vi "FixJKIHelper.vi"() -> ()   [LabVIEW 2017]
uses:
  _Support/Common/Format Timestamp.vi
  _Shared/CSM Shared.lvlib
  _csmDoc/csmdoc.lvlib
  Communicable State Machine.lvlib
  user32.dll
panel:
  out "String Cache":string
  in  "Bottom Right":string
  in  "Bottom Left":string
  out "2D Picture":picture
  in  "Error in":errorcluster caption="error in (no error)"
  out "Listbox":i32(listbox)
  in  "Progress Bar":u8(slide) scale=-1.0..291.0
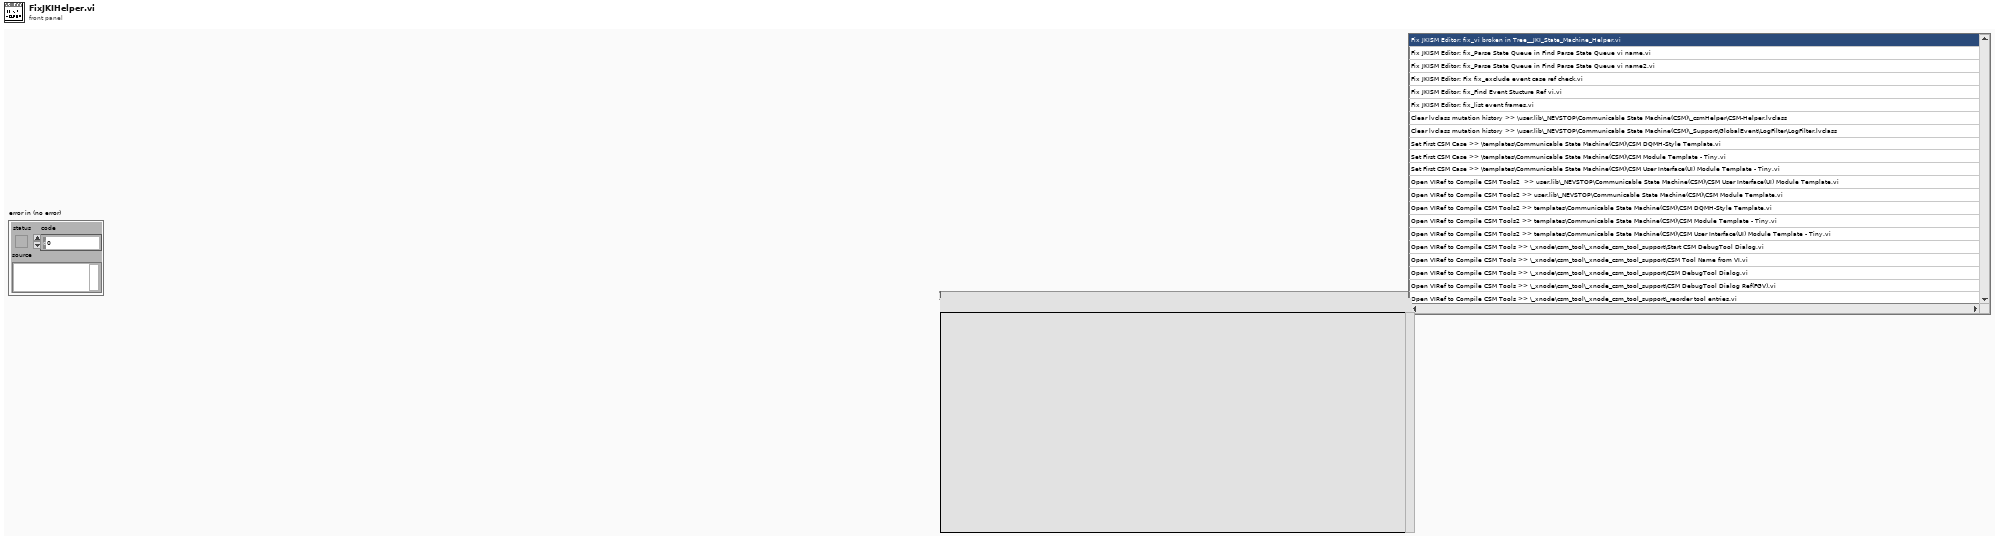
[diagram p1: front panel]
types:
  T1 = enum32{"Invalid", "Standard", "Closed", "Hidden", "Minimized", "Maximized"}
  T2 = enum32{"invalid app kind", "Development System", "Run Time System", "Student Edition", "Embedded LabVIEW", "Evaluation", "Custom"}
  T3 = cluster{"Core":cluster{"Current VI Reference":refnum<vi>, "Close Panel on Exit?":bool}, "Listbox Symbols":i32[], "Listbox Index":i32, "_JKI State Machine Helper VIs":path[], "CSM Templates":path[], "CSM lvclass":path[], "_JKI State Machine Helper Folders":path[], "Actions":string[], "LangID":string, "DescMap":variant, "NoteMap":variant, "Polish":cluster{"Version":refnum<vi>, "Action":refnum<vi>, "Progress Bar":refnum<vi>, "2D Picture":refnum<vi>, "Hold":bool, "Slides":picture[]}}
  T4 = cluster{"Version":refnum<vi>, "Action":refnum<vi>, "Progress Bar":refnum<vi>, "2D Picture":refnum<vi>, "Hold":bool, "Slides":picture[]}
  T5 = cluster{"Current VI Reference":refnum<vi>, "Close Panel on Exit?":bool}
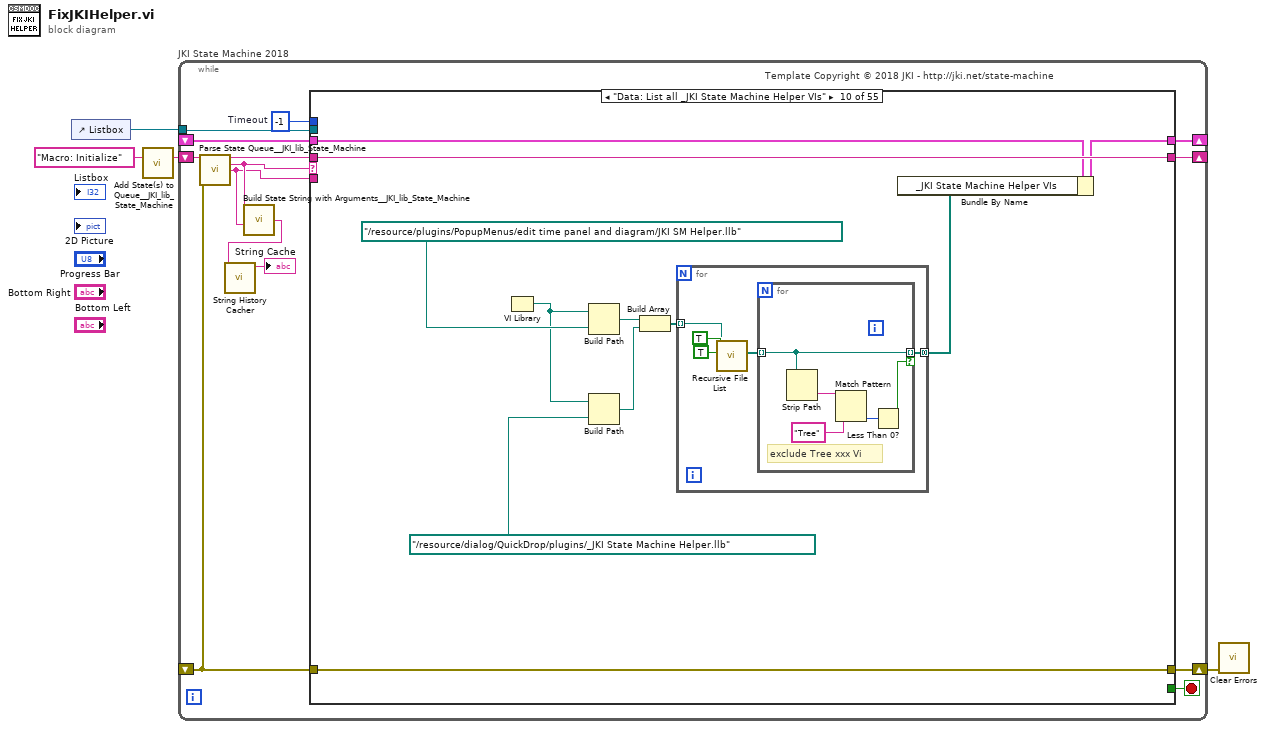
[diagram p0: block diagram]
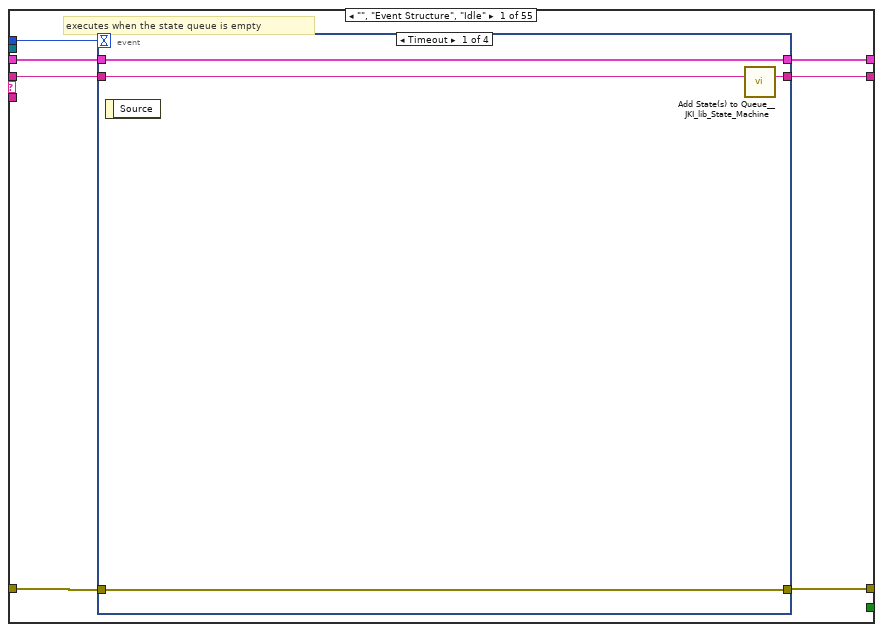
[diagram p2: hidden frame]
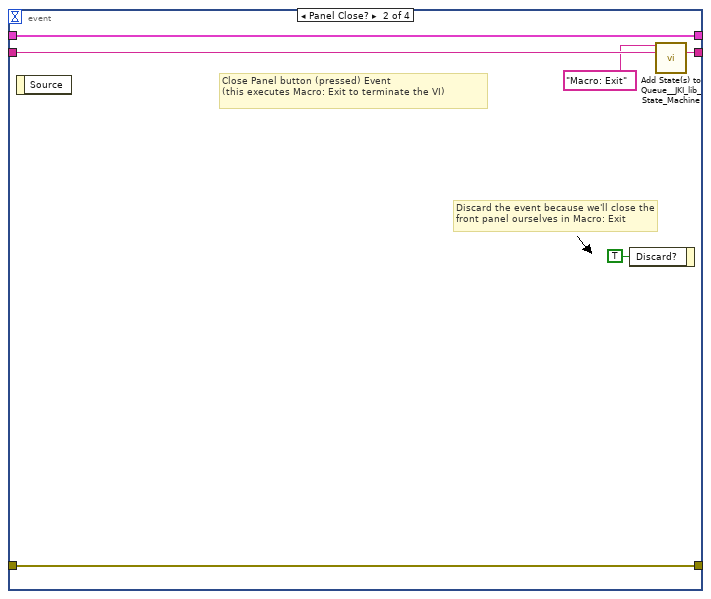
[diagram p3: hidden frame]
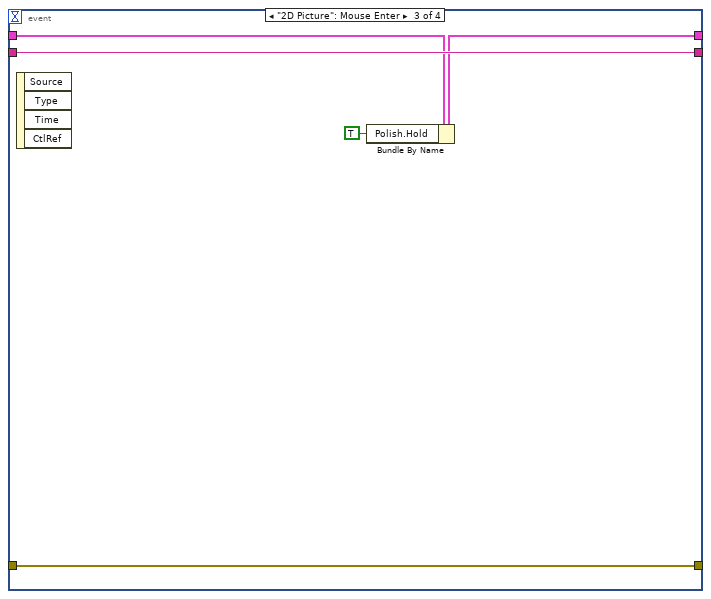
[diagram p4: hidden frame]
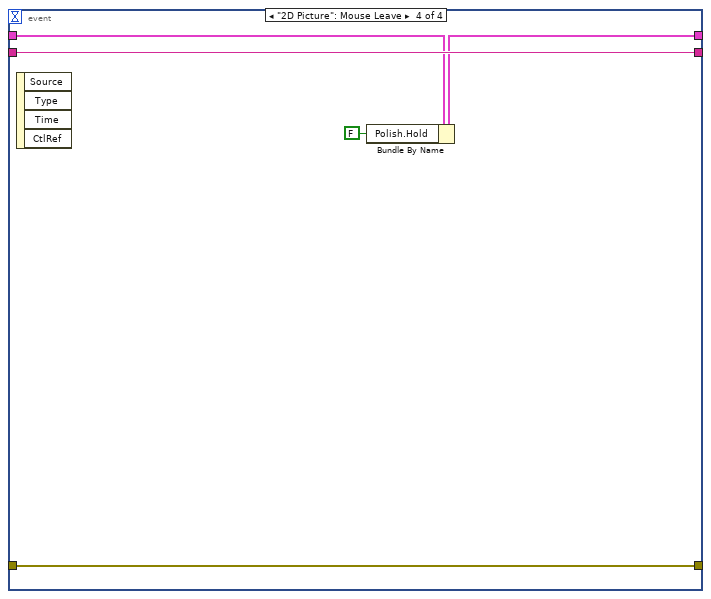
[diagram p5: hidden frame]
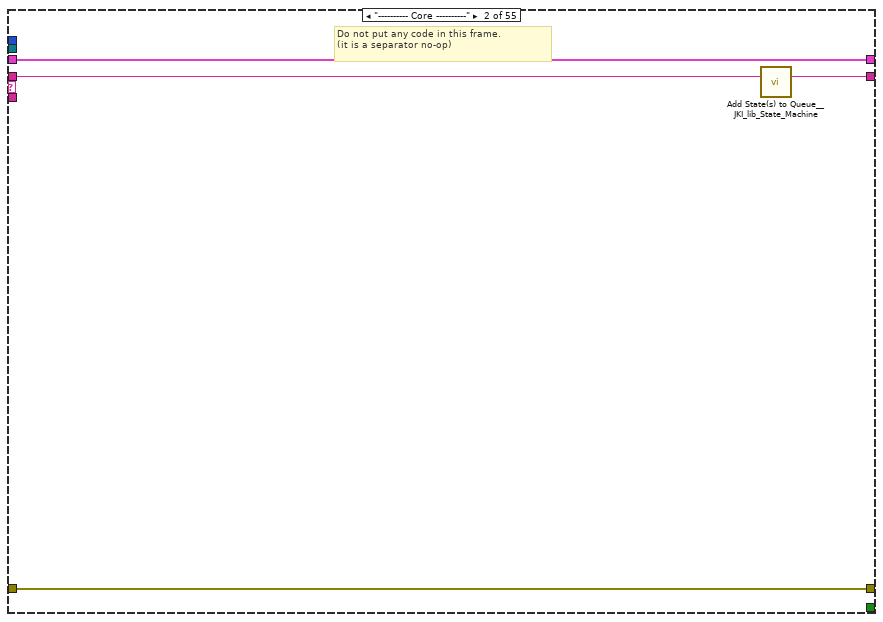
[diagram p6: hidden frame]
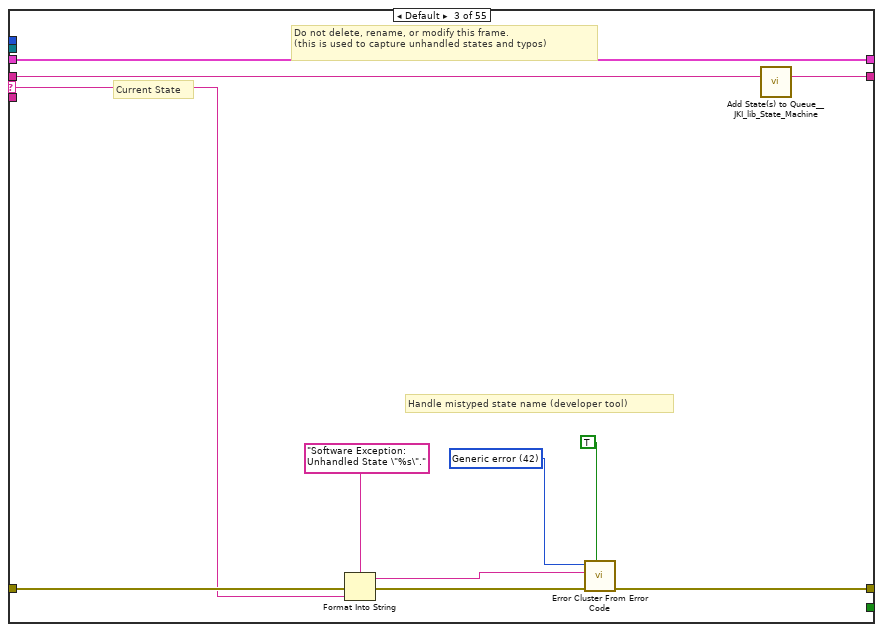
[diagram p7: hidden frame]
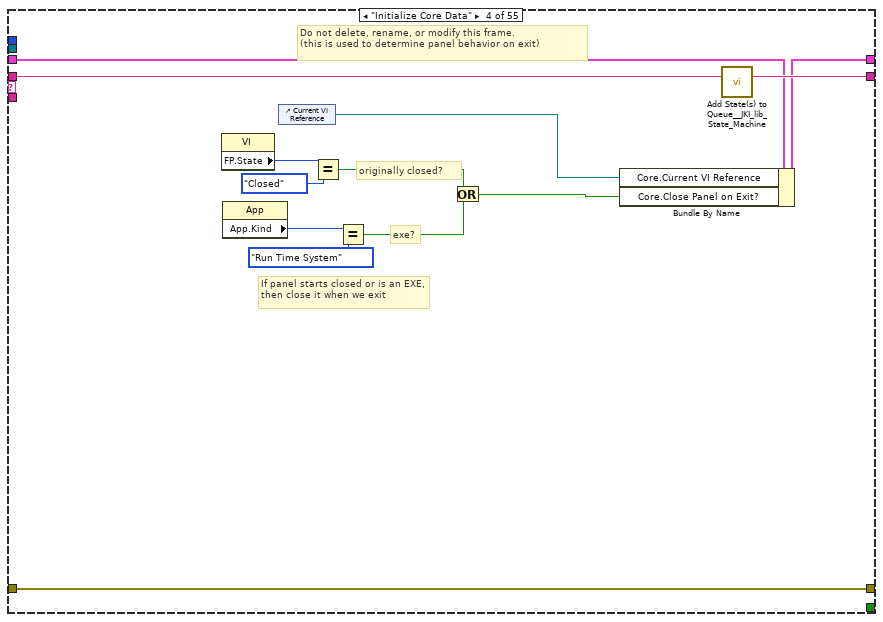
[diagram p8: hidden frame]
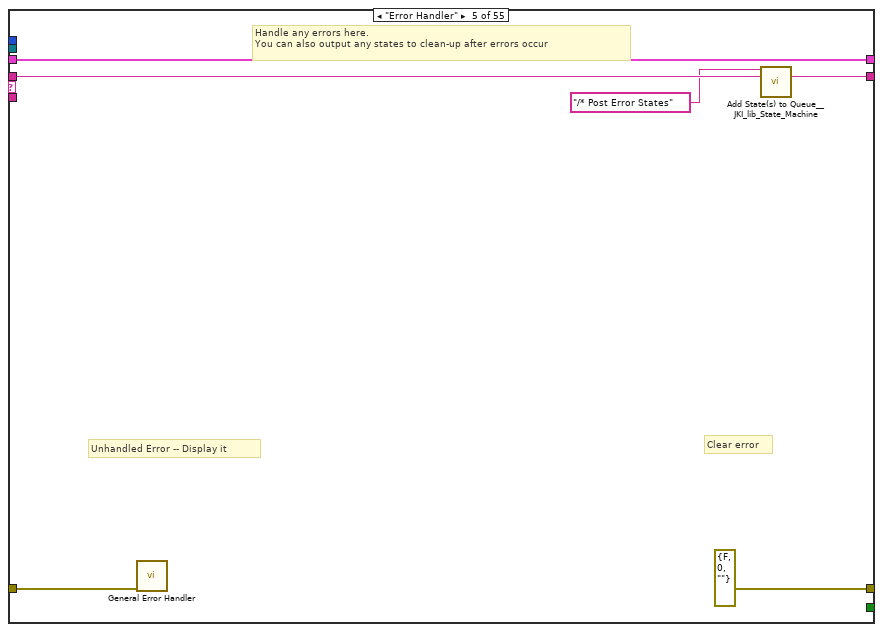
[diagram p9: hidden frame]
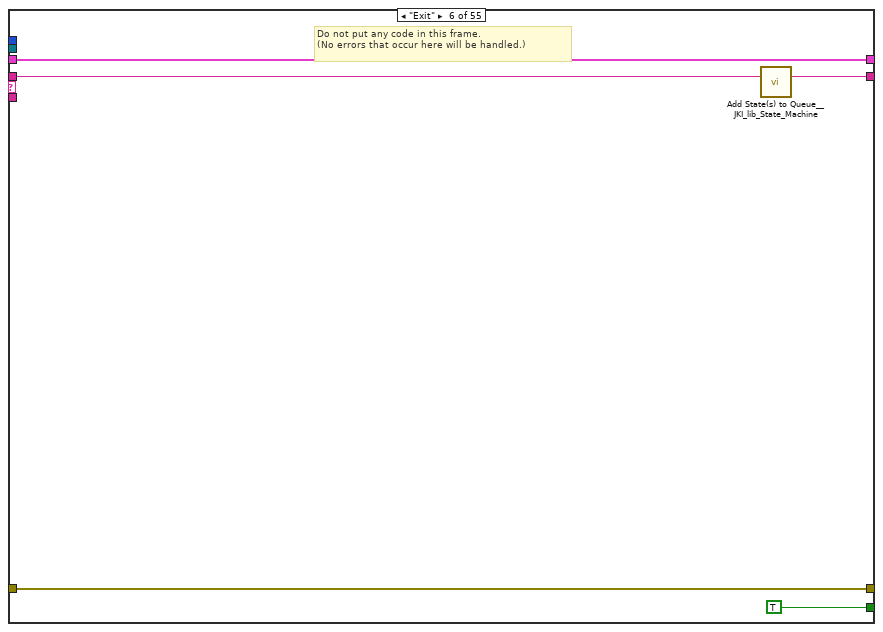
[diagram p10: hidden frame]
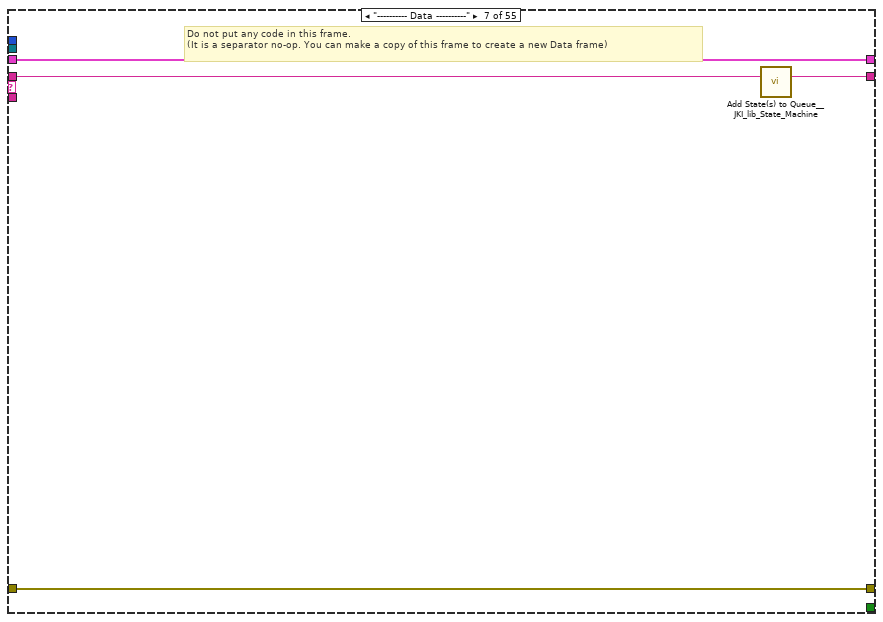
[diagram p11: hidden frame]
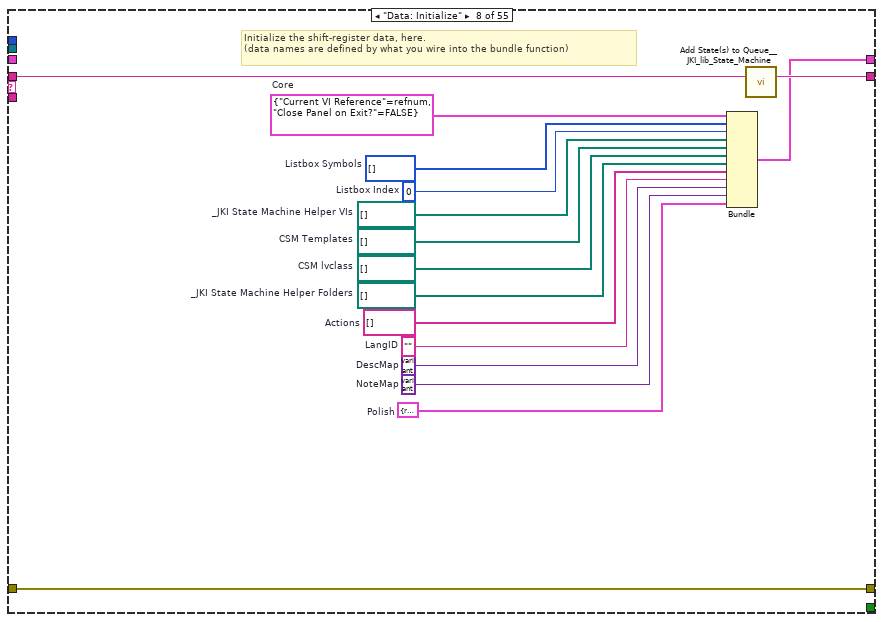
[diagram p12: hidden frame]
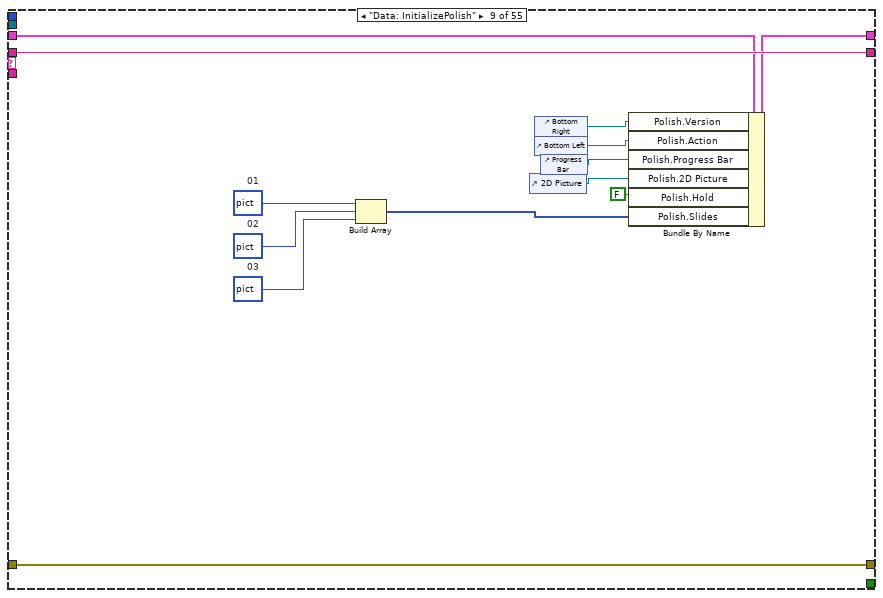
[diagram p13: hidden frame]
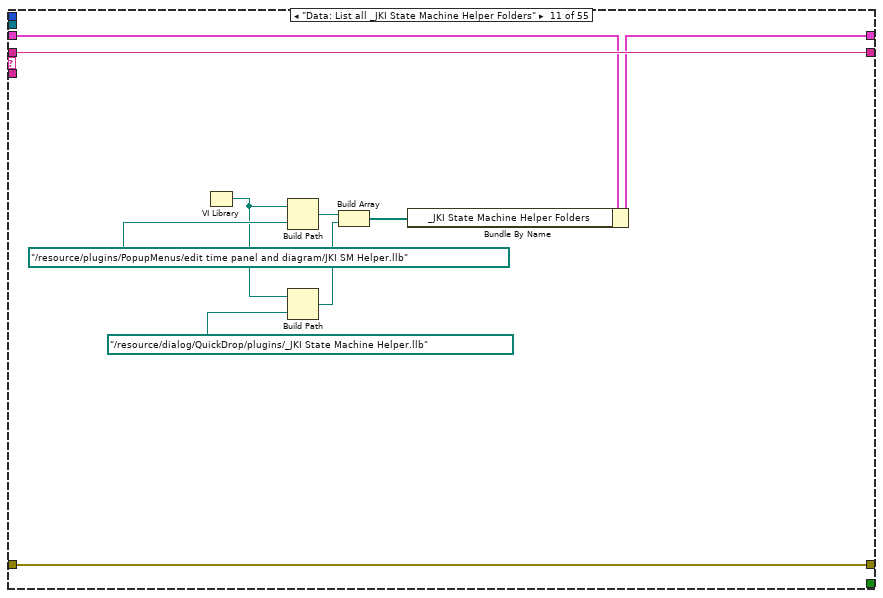
[diagram p14: hidden frame]
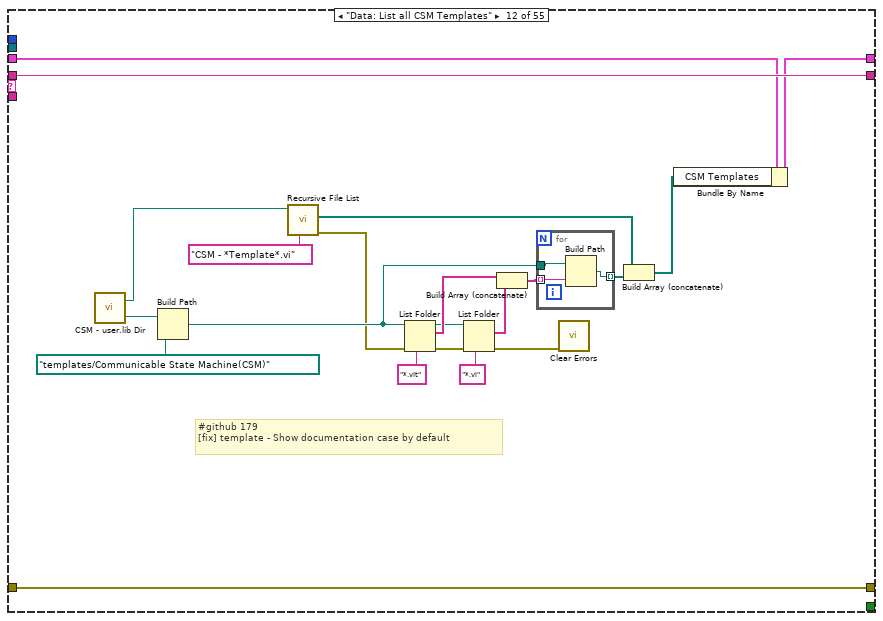
[diagram p15: hidden frame]
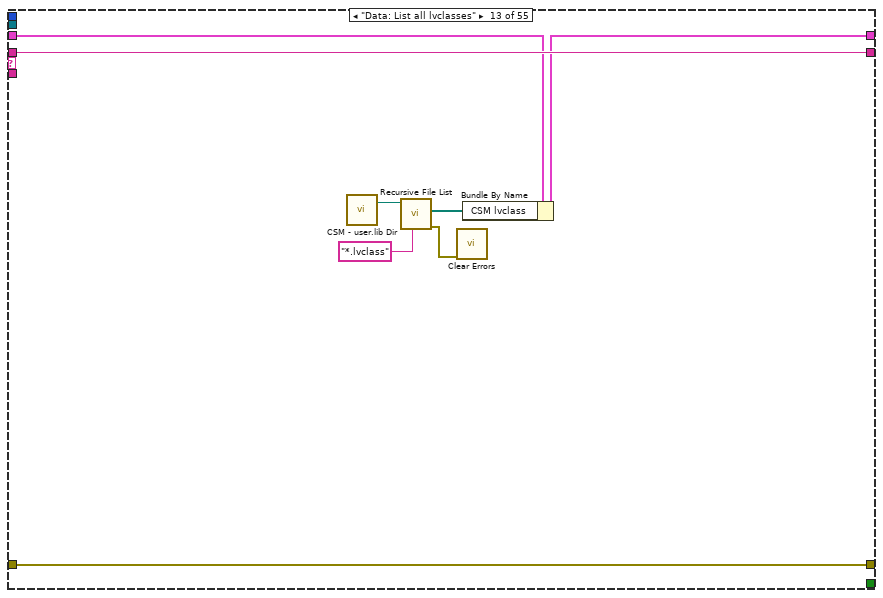
[diagram p16: hidden frame]
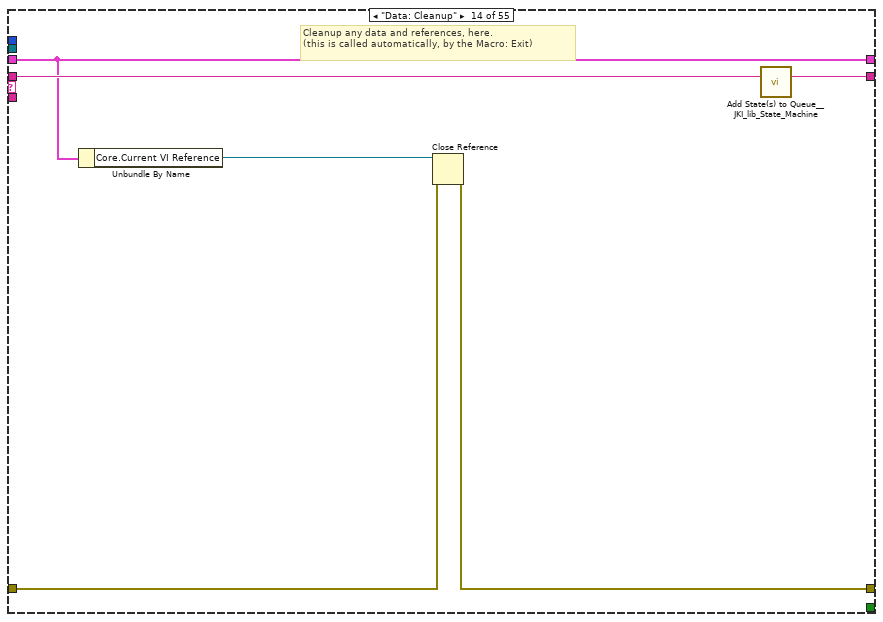
[diagram p17: hidden frame]
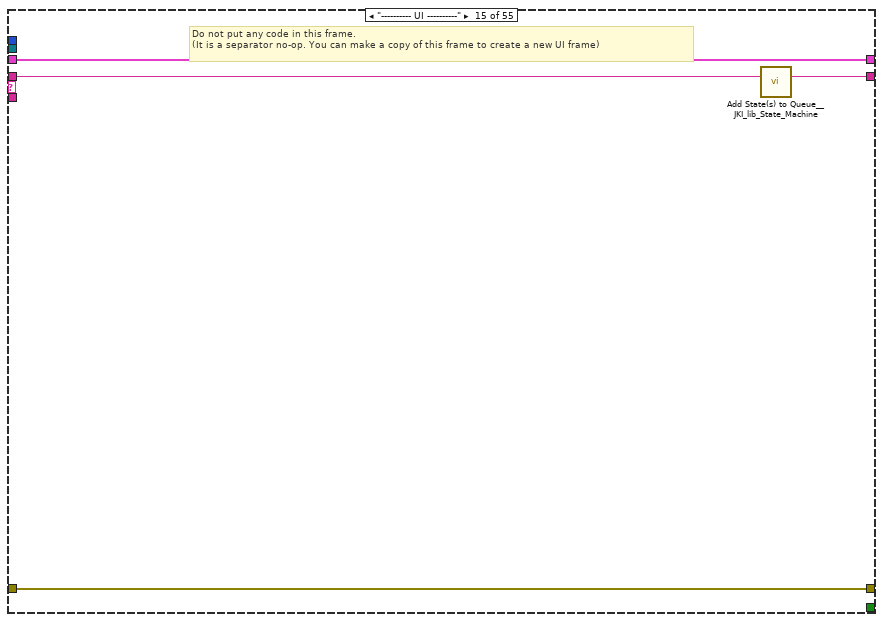
[diagram p18: hidden frame]
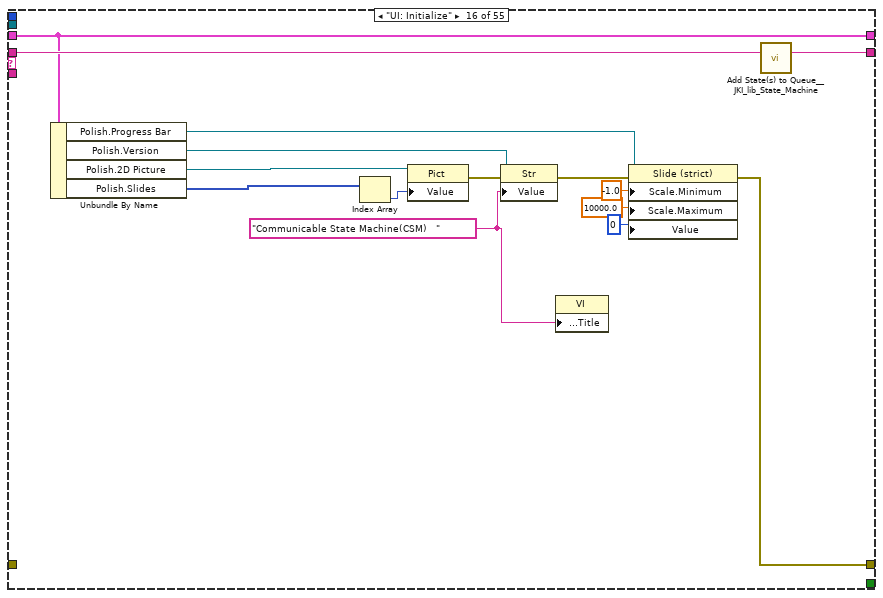
[diagram p19: hidden frame]
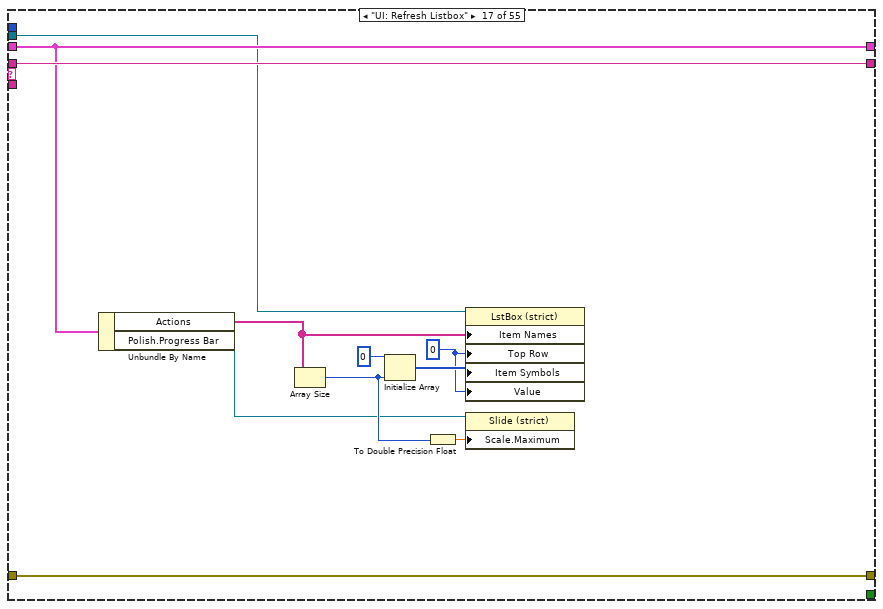
[diagram p20: hidden frame]
diagram:
  n1 = control-ref of="Listbox"() -> (w2:refnum<vi>)
  n2 = call <vilib>:"Add State(s) to Queue__JKI_lib_State_Machine.vi"("State(s) in (\"\")"="Macro: Initialize") -> ("States Out"=w4:string)  [unwired: 14 in]
  n3 = while "JKI State Machine 2018" {
    shift-right: [w13] -> _
    shift-left: _ -> [w12]
    shift-right: [w16] -> w1
    shift-left: _ -> [w10]
    shift-right: [w15] -> _
    shift-left: w4 -> [w17]
    tunnel: w2 -> [w9]
    stop <- w14 stop-if-true
    w11 = -1  # Timeout
    # "Template Copyright © 2018 JKI - http://jki.net/state-machine"
    n4 = call <vilib>:"Parse State Queue__JKI_lib_State_Machine.vi"("State Queue"=w17, "Error In (no error)"=w10) -> ("Remaining States"=w18:string, "Current State"=w7:string, "Arguments"=w6:string)  [unwired: 11 in]
    n5 = call <vilib>:"Build State String with Arguments__JKI_lib_State_Machine.vi"("Arguments (\"\")"=w6, "State"=w7) -> ("State with Arguments"=w5:string)  [unwired: 4 in]
    n6 = call "String History Cacher.vi"("String"=w5) -> ("String Cache"=→"String Cache":string)  [unwired: 10 in]
    n7 = case shown="\"Data: List all _JKI State Machine Helper VIs\"" w7 {
      selector: w7 -> [_ _ w50 _ _ _ _ _ _ _ _ _ _ _ _ _ _ _ _ _ _ _ _ _ _ _ _ _ _ _ _ _ _ _ _ _ _ _ _ _ _ _ _ _ _ _ _ _ _ _ _ _ _ _ _]
      tunnel: w18 -> [w25 w49 w54 w73 w79 w84 w88 w104 w116 w128 w148 w168 w179 w186 w190 w205 w215 w222 w229 w263 w330 w370 w375 w377 w391 w415 w421 w427 w438 w440 w451 w465 w474 w491 w507 w522 w536 w549 w551 w573 w585 w590 w595 w600 w605 w610 w615 w626 w639 w670 w700 w722 w740 w748 w757]
      tunnel: w6 -> [_ _ _ _ _ _ _ _ _ _ _ _ _ _ _ _ _ w217 _ w257 _ _ _ _ _ _ _ _ _ _ _ _ _ _ _ w521 _ _ w554 w567 w579 _ _ _ _ _ _ w620 w634 w663 w694 _ _ _ w754]
      tunnel: w12 -> [w23 w46 w52 w66 w76 w82 w85 _ w115 w127 w147 w167 w178 w181 w187 w202 w212 w220 w227 w259 w339 w367 w372 w380 w393 w417 w423 w426 w435 w439 w449 w463 w472 w490 w505 w519 w534 w546 w564 w576 w587 w592 w597 w602 w607 w612 w617 w629 w641 w672 w702 w730 w744 w751 w760]
      tunnel: [w22 w47 w56 w70 errorcluster {"status"=FALSE, "code"=0, "source"=""} ("error out") w81 w86 w101 w117 w118 w140 w169 w180 w182 w188 w192 w216 w218 w228 w260 w357 w368 w373 w381 w394 w418 w424 w428 w436 w441 w447 w464 w470 w488 w503 w515 w533 w547 w565 w577 w588 w593 w598 w603 w608 w613 w618 w631 w642 w673 w703 w731 w745 "Error in" w759] -> w16
      tunnel: w10 -> [w21 w47 w55 w70 w75 w81 w86 w101 w117 w118 w140 w169 w180 w183 w188 _ w216 w219 _ w261 w357 w368 w373 w381 w394 w418 w424 w428 w436 w441 w447 w464 w470 w488 w503 w515 w533 w547 w565 w577 w588 w593 w598 w603 w608 w613 w618 w631 w642 w673 w703 w731 w745 _ _]
      tunnel: [w24 w48 w53 w72 w78 w83 w87 w103 w116 w128 w148 w168 w179 w185 w189 w204 w215 w221 w229 w262 w331 w369 w374 w378 w392 w416 w422 w427 w437 w440 w451 w465 w474 w491 w507 w522 w536 w548 w552 w574 w586 w591 w596 w601 w606 w611 w616 w627 w640 w671 w701 w723 w741 w749 w758] -> w15
      tunnel: [_ _ _ _ _ TRUE _ _ _ _ _ _ _ _ _ _ _ _ _ _ _ _ _ _ _ _ _ _ _ _ _ _ _ _ _ _ _ _ _ _ _ _ _ _ _ _ _ _ _ _ _ _ _ _ _] -> w14
      tunnel: [w20 w46 w52 w71 w76 w82 w85 w102 w114 w120 w141 w150 w175 w181 w187 w202 w212 w220 w227 w259 w339 w367 w372 w380 w393 w417 w423 w426 w435 w439 w444 w462 w468 w485 w501 w518 w532 w546 w564 w576 w587 w592 w597 w602 w607 w612 w617 w629 w641 w672 w702 w730 w743 w750 w760] -> w13
      tunnel: w11 -> [w19 _ _ _ _ _ _ _ _ _ _ _ _ _ _ _ _ _ _ _ _ _ _ _ _ _ _ _ _ _ _ _ _ _ _ _ _ _ _ _ _ _ _ _ _ _ _ _ _ _ _ _ _ _ _]
      tunnel: w9 -> [_ _ _ _ _ _ _ _ _ _ _ _ _ _ _ _ w211 _ _ _ w346 _ _ _ _ _ _ _ _ _ _ _ _ _ _ _ _ _ _ _ _ _ _ _ _ _ _ _ _ _ _ _ _ _ _]
      frame "", "Event Structure", "Idle" {
        # "executes when the state queue is empty"
        n8 = event shown="[0] Timeout" {
          selector: _ -> [_ _ _ _]
          dyn-events: _ -> [_ _ _ _]
          timeout: w19 -> [_ _ _ _]
          tunnel: w25 -> [w29 w35 w40 w45]
          tunnel: [w28 w34 w40 w45] -> w24
          tunnel: w23 -> [w26 w32 w38 w43]
          tunnel: [w27 w33 w39 w44] -> w22
          tunnel: w21 -> [w27 w33 w39 w44]
          tunnel: [w26 w32 w36 w41] -> w20
          event Timeout {
            n9 = event-data() -> ()  [unwired: 1 in, 1 out]
            n10 = call <vilib>:"Add State(s) to Queue__JKI_lib_State_Machine.vi"("State(s) in (\"\")"=w29) -> ("States Out"=w28:string)  [unwired: 14 in]
          }
          event Panel Close? {
            # "Discard the event because we'll close the front panel ourselves in Macro: Exit"
            # "Close Panel button (pressed) Event\n(this executes Macro: Exit to terminate the VI)"
            n11 = event-data() -> ()  [unwired: 1 in, 1 out]
            n12 = event-data("Discard?"=TRUE) -> ()  [unwired: 1 in, 1 out]
            n13 = call <vilib>:"Add State(s) to Queue__JKI_lib_State_Machine.vi"("State(s) in Front (\"\")"="Macro: Exit", "State(s) in (\"\")"=w35) -> ("States Out"=w34:string)  [unwired: 13 in]
          }
          event "2D Picture": Mouse Enter {
            n14 = event-data() -> ()  [unwired: 1 in, 4 out]
            n15 = Bundle By Name(cluster=w38, "Polish.Hold"=TRUE) -> (w36:T3)
          }
          event "2D Picture": Mouse Leave {
            n16 = event-data() -> ()  [unwired: 1 in, 4 out]
            n17 = Bundle By Name(cluster=w43, "Polish.Hold"=FALSE) -> (w41:T3)
          }
        }
      }
      frame "---------- Core ----------" {
        # "Do not put any code in this frame.\n(it is a separator no-op)"
        n18 = call <vilib>:"Add State(s) to Queue__JKI_lib_State_Machine.vi"("State(s) in (\"\")"=w49) -> ("States Out"=w48:string)  [unwired: 14 in]
      }
      frame Default {
        w59 = 42 items=["No error", "Argument error", "Memory is full", "Out of zone", "End of file", "File already open", "Generic file I/O error", "File not found", "File permission error", "Disk is full", "Duplicate path", "Too many files open", "System feature not enabled", "Resource file not found", "Cannot add resource", "Resource not found", "Image not found", "Image memory error", "Pen does not exist", "Config type invalid", "Config token not found", "Config parse error", "Config memory error", "Bad external code format", "Bad external code offset", "External code not present", "Null window", "Destroy window error", "Null menu", "Print aborted", "Bad print record", "Print driver error", "Windows error during printing", "Memory error during printing", "Print dialog error", "Generic print error", "Invalid device refnum", "Device not found", "Device parameter error", "Device unit error", "Cannot open device", "Device call aborted", "Generic error", "Cancelled by user", "Object ID too low", "Object ID too high", "Object not in heap", "Unknown heap", "Unknown object (invalid DefProc)", "Unknown object (DefProc not in table)", "Message out of range", "Invalid (null) method", "Unknown message", "Manager call not supported", "Bad address", "Network operation in progress", "Network operation timed out", "Connection is busy", "Network attribute not supported", "Network error", "Address in use", "System out of memory", "Connection aborted", "Connection refused", "Not connected", "Already connected", "Connection closed", "Initialization error (interapplication manager)", "Bad occurrence", "Wait on unbound occurrence handler", "Occurrence queue overflow", "Datalog type conflict", "Unused", "Unrecognized type (interapplication manager)", "Memory corrupt", "Failed to make temporary DLL", "Old CIN version", "Drag socket not found", "Failed to load drop-object", "Failed to register OLE object", "Failed to release OLE object", "Format specifier type mismatch", "Unknown format specifier", "Too few format specifiers", "Too many format specifiers", "Scan failed", "Newer CIN version", "Error converting to variant", "Runtime menu error", "Password tampered", "Variant attribute not found", "Incompatible variant data type", "Event data is not available", "Event Store is not present", "Occurrence is not found", "Event Queue is not created", "Event info is not available", "Refnum passed is NULL", "Error retrieving Class GUID", "Error retrieving CoClass GUID", "Error retrieving TypeLib GUID.", "Bad built application magic bytes.", "Specific driver is different from the specific driver associated with the Logical Name.", "There is no session opened to the class driver.", "Max Error", "MAX - Error with config objects", "MAX - Error loading configuration", "MAX - Group not supported"]
        # "Current State"
        # "Do not delete, rename, or modify this frame.\n(this is used to capture unhandled states and typos)"
        # "Handle mistyped state name (developer tool)"
        n19 = Format Into String(format string="Software Exception: Unhandled State \"%s\"." ("message"), error in=w55, w50) -> (resulting string=w58:string, error out=w57:errorcluster)  [unwired: 1 in]
        n20 = call <vilib>:"Error Cluster From Error Code.vi"("show call chain? (False)"=TRUE, "error in (no error)"=w57, "error message (\"\")"=w58, "error code (0)"=w59) -> ("error out"=w56:errorcluster)  [unwired: 5 in]
        n21 = call <vilib>:"Add State(s) to Queue__JKI_lib_State_Machine.vi"("State(s) in (\"\")"=w54) -> ("States Out"=w53:string)  [unwired: 14 in]
      }
      frame "Initialize Core Data" {
        # "Do not delete, rename, or modify this frame.\n(this is used to determine panel behavior on exit)"
        # "originally closed?"
        # "exe?"
        # "If panel starts closed or is an EXE, then close it when we exit"
        n22 = property class="VI"() -> ("FP.State"=w63:T1)  [unwired: 2 in, 2 out]
        n23 = property class="App"() -> ("App.Kind"=w69:T2)  [unwired: 2 in, 2 out]
        n24 = control-ref of="Current VI Reference"() -> (w64:refnum<vi>)
        n25 = Equal?(x=w63, y=T1."Closed" ("Front Panel Window:State")) -> (x = y?=w61:bool)
        n26 = Equal?(x=w69, y=T2."Run Time System" ("Application:Kind")) -> (x = y?=w67:bool)
        n27 = Or(x=w61, y=w67) -> (x .or. y?=w65:bool)
        n28 = Bundle By Name(cluster=w66, "Core.Current VI Reference"=w64, "Core.Close Panel on Exit?"=w65) -> (w71:T3)
        n29 = call <vilib>:"Add State(s) to Queue__JKI_lib_State_Machine.vi"("State(s) in (\"\")"=w73) -> ("States Out"=w72:string)  [unwired: 14 in]
      }
      frame "Error Handler" {
        # "Unhandled Error -- Display it"
        # "Handle any errors here.\nYou can also output any states to clean-up after errors occur"
        # "Clear error"
        n30 = call <vilib>:"General Error Handler.vi"("error in (no error)"=w75) -> ()  [unwired: 10 in, 5 out]
        n31 = call <vilib>:"Add State(s) to Queue__JKI_lib_State_Machine.vi"("State(s) in Front (\"\")"="/* Post Error States", "State(s) in (\"\")"=w79) -> ("States Out"=w78:string)  [unwired: 13 in]
      }
      frame "Exit" {
        # "Do not put any code in this frame.\n(No errors that occur here will be handled.)"
        n32 = call <vilib>:"Add State(s) to Queue__JKI_lib_State_Machine.vi"("State(s) in (\"\")"=w84) -> ("States Out"=w83:string)  [unwired: 14 in]
      }
      frame "---------- Data ----------" {
        # "Do not put any code in this frame.\n(It is a separator no-op. You can make a copy of this frame to create a new Data frame)"
        n33 = call <vilib>:"Add State(s) to Queue__JKI_lib_State_Machine.vi"("State(s) in (\"\")"=w88) -> ("States Out"=w87:string)  [unwired: 14 in]
      }
      frame "Data: Initialize" {
        w89 = T4 {"Version"=refnum, "Action"=refnum, "Progress Bar"=refnum, "2D Picture"=refnum, "Hold"=TRUE, "Slides"=[]}  # Polish
        w90 = variant  # NoteMap
        w91 = variant  # DescMap
        w92 = ""  # LangID
        w93 = string[] []  # Actions
        w94 = path[] []  # _JKI State Machine Helper Folders
        w95 = path[] []  # CSM lvclass
        w96 = i32[] []  # Listbox Symbols
        w97 = 0  # Listbox Index
        w98 = path[] []  # CSM Templates
        w99 = path[] []  # _JKI State Machine Helper VIs
        w100 = T5 {"Current VI Reference"=refnum, "Close Panel on Exit?"=FALSE}  # Core
        # "Initialize the shift-register data, here.\n(data names are defined by what you wire into the bundle function)"
        n34 = Bundle("Core"=w100, "Listbox Symbols"=w96, "Listbox Index"=w97, "_JKI State Machine Helper VIs"=w99, "CSM Templates"=w98, "CSM lvclass"=w95, "_JKI State Machine Helper Folders"=w94, "Actions"=w93, "LangID"=w92, "DescMap"=w91, "NoteMap"=w90, "Polish"=w89) -> (w102:T3)  [unwired: 1 in]
        n35 = call <vilib>:"Add State(s) to Queue__JKI_lib_State_Machine.vi"("State(s) in (\"\")"=w104) -> ("States Out"=w103:string)  [unwired: 14 in]
      }
      frame "Data: InitializePolish" {
        w105 = picture bytes[1036830]  # 03
        w106 = picture bytes[1036830]  # 02
        w107 = picture bytes[1036830]  # 01
        n36 = Build Array(w107, w106, w105) -> (w110:picture[])
        n37 = control-ref of="2D Picture"() -> (w112:refnum<vi>)
        n38 = control-ref of="Bottom Right"() -> (w109:refnum<vi>)
        n39 = control-ref of="Bottom Left"() -> (w108:refnum<vi>)
        n40 = control-ref of="Progress Bar"() -> (w113:refnum<vi>)
        n41 = Bundle By Name(cluster=w115, "Polish.Version"=w109, "Polish.Action"=w108, "Polish.Progress Bar"=w113, "Polish.2D Picture"=w112, "Polish.Hold"=FALSE, "Polish.Slides"=w110) -> (w114:T3)
      }
      frame "Data: List all _JKI State Machine Helper VIs" {
        n42 = VI Library() -> (path=w125:path)
        n43 = Build Path(base path=w125, name or relative path=path "../resource/plugins/PopupMenus/edit time panel and diagram/JKI SM Helper.llb") -> (appended path=w123:path)
        n44 = Build Path(base path=w125, name or relative path=path "../resource/dialog/QuickDrop/plugins/_JKI State Machine Helper.llb") -> (appended path=w121:path)
        n45 = Build Array(w123, w121) -> (w122:path[])
        n46 = for {
          tunnel: w122 -> [w131] mode=indexing
          tunnel: [w129] -> w119 mode=concatenating
          n47 = call <vilib>:"Recursive File List.vi"("Continue Recursing on Error? (F)"=TRUE, "Treat LLBs as Folders?"=TRUE, "Folder Path"=w131) -> ("All Files in Dir"=w130:path[])  [unwired: 4 in, 4 out]
          n48 = for {
            tunnel: w130 -> [w135] mode=indexing
            tunnel: [w135] -> w129 mode=indexing if=w134
            # "exclude Tree xxx Vi"
            n49 = Strip Path(path=w135) -> (name=w138:string)  [unwired: 1 out]
            n50 = Match Pattern(string=w138, regular expression="Tree") -> (offset past match=w136:i32)  [unwired: 1 in, 3 out]
            n51 = Less Than 0?(x=w136) -> (x < 0?=w134:bool)
          }
        }
        n52 = Bundle By Name(cluster=w127, "_JKI State Machine Helper VIs"=w119) -> (w120:T3)
      }
      frame "Data: List all _JKI State Machine Helper Folders" {
        n53 = VI Library() -> (path=w145:path)
        n54 = Build Path(base path=w145, name or relative path=path "../resource/plugins/PopupMenus/edit time panel and diagram/JKI SM Helper.llb") -> (appended path=w143:path)
        n55 = Build Path(base path=w145, name or relative path=path "../resource/dialog/QuickDrop/plugins/_JKI State Machine Helper.llb") -> (appended path=w142:path)
        n56 = Build Array(w143, w142) -> (w139:path[])
        n57 = Bundle By Name(cluster=w147, "_JKI State Machine Helper Folders"=w139) -> (w141:T3)
      }
      frame "Data: List all CSM Templates" {
        # "#github 179\n[fix] template - Show documentation case by default"
        n58 = call "CSM - user.lib Dir.vi"() -> ("<LabVIEW>"=w157:path, "csm_user.lib_dir"=w159:path)  [unwired: 2 in]
        n59 = Build Path(base path=w157, name or relative path=path "templates/Communicable State Machine(CSM)") -> (appended path=w166:path)
        n60 = call <vilib>:"Recursive File List.vi"("pattern"="CSM - *Template*.vi" ("name or relative path"), "Folder Path"=w159) -> ("error out"=w160:errorcluster, "All Files in Dir"=w161:path[])  [unwired: 5 in, 3 out]
        n61 = List Folder(path=w166, pattern="*.vit", error in=w160) -> (path out=w153:path, filenames=w162:string[], error out=w155:errorcluster)  [unwired: 1 in, 1 out]
        n62 = List Folder(path=w153, pattern="*.vi", error in=w155) -> (filenames=w163:string[], error out=w156:errorcluster)  [unwired: 1 in, 2 out]
        n63 = Build Array (concatenate)(w162, w163) -> (w164:string[])
        n64 = for {
          tunnel: w164 -> [w172] mode=indexing
          tunnel: [w171] -> w165 mode=indexing
          tunnel: w166 -> [w170]
          n65 = Build Path(base path=w170, name or relative path=w172) -> (appended path=w171:path)
        }
        n66 = call <vilib>:"Clear Errors.vi"("error in (no error)"=w156) -> ()  [unwired: 5 in, 2 out]
        n67 = Build Array (concatenate)(w161, w165) -> (w149:path[])
        n68 = Bundle By Name(cluster=w167, "CSM Templates"=w149) -> (w150:T3)
      }
      frame "Data: List all lvclasses" {
        n69 = call "CSM - user.lib Dir.vi"() -> ("csm_user.lib_dir"=w177:path)  [unwired: 2 in, 1 out]
        n70 = call <vilib>:"Recursive File List.vi"("pattern"="*.lvclass", "Folder Path"=w177) -> ("error out"=w173:errorcluster, "All Files in Dir"=w174:path[])  [unwired: 5 in, 3 out]
        n71 = call <vilib>:"Clear Errors.vi"("error in (no error)"=w173) -> ()  [unwired: 5 in, 2 out]
        n72 = Bundle By Name(cluster=w178, "CSM lvclass"=w174) -> (w175:T3)
      }
      frame "Data: Cleanup" {
        # "Cleanup any data and references, here.\n(this is called automatically, by the Macro: Exit)"
        n73 = Unbundle By Name(w181) -> ("Core.Current VI Reference"=w184:refnum<vi>)
        n74 = Close Reference(reference=w184, error in (no error)=w183) -> (error out=w182:errorcluster)
        n75 = call <vilib>:"Add State(s) to Queue__JKI_lib_State_Machine.vi"("State(s) in (\"\")"=w186) -> ("States Out"=w185:string)  [unwired: 14 in]
      }
      frame "---------- UI ----------" {
        # "Do not put any code in this frame.\n(It is a separator no-op. You can make a copy of this frame to create a new UI frame)"
        n76 = call <vilib>:"Add State(s) to Queue__JKI_lib_State_Machine.vi"("State(s) in (\"\")"=w190) -> ("States Out"=w189:string)  [unwired: 14 in]
      }
      frame "UI: Initialize" {
        w191 = "Communicable State Machine(CSM)   " ("Value")
        n77 = Unbundle By Name(w202) -> ("Polish.Progress Bar"=w196:refnum<vi>, "Polish.Version"=w199:refnum<vi>, "Polish.2D Picture"=w201:refnum<vi>, "Polish.Slides"=w203:picture[])
        n78 = Index Array(array=w203) -> (element=w200:picture)  [unwired: 1 in]
        n79 = property class="Pict"(reference=w201, "Value"=w200) -> (error out=w198:errorcluster)  [unwired: 1 in, 1 out]
        n80 = property class="Str"(reference=w199, error in=w198, "Value"=w191) -> (error out=w197:errorcluster)  [unwired: 1 out]
        n81 = property class="VI"("Front Panel.Title"=w191) -> ()  [unwired: 2 in, 2 out]
        n82 = property class="Slide (strict)"(reference=w196, error in=w197, "Scale.Minimum"=-1.0 ("Scale.Range:Minimum"), "Scale.Maximum"=10000.0 ("Scale.Range:Maximum"), "Value"=u8 0) -> (error out=w192:errorcluster)  [unwired: 1 out]
        n83 = call <vilib>:"Add State(s) to Queue__JKI_lib_State_Machine.vi"("State(s) in (\"\")"=w205) -> ("States Out"=w204:string)  [unwired: 14 in]
      }
      frame "UI: Refresh Listbox" {
        w210 = 0 ("Top Row")
        n84 = Unbundle By Name(w212) -> ("Actions"=w208:string[], "Polish.Progress Bar"=w206:refnum<vi>)
        n85 = Array Size(array=w208) -> (size(s)=w207:i32)
        n86 = Initialize Array(0 ("Top Row"), w207) -> (w213:i32[])
        n87 = To Double Precision Float(number=w207) -> (double precision float=w209:dbl)
        n88 = property on="Property Node" class="LstBox (strict)"(reference=w211, "Item Names"=w208, "Top Row"=w210, "Item Symbols"=w213, "Value"=w210) -> ()  [unwired: 1 in, 2 out]
        n89 = property class="Slide (strict)"(reference=w206, "Scale.Maximum"=w209) -> ()  [unwired: 1 in, 2 out]
      }
      frame "UI: Cursor Set" {
        # "Argument"
        # "Set and Unset Cursor Busy.\n(Usage: \"UI: Cursor Set >> Busy|Idle\")"
        n90 = case shown="\"Idle\", Default" w217 {
          tunnel: w219 -> [w224 w226]
          tunnel: [w223 w225] -> w218
          frame "Idle", Default {
            n91 = call <vilib>:"Unset Busy.vi"("error in (no error)"=w224) -> ("error out"=w223:errorcluster)  [unwired: 10 in]
          }
          frame "Busy" {
            n92 = call <vilib>:"Set Busy.vi"("error in (no error)"=w226) -> ("error out"=w225:errorcluster)  [unwired: 9 in, 1 out]
          }
        }
        n93 = call <vilib>:"Add State(s) to Queue__JKI_lib_State_Machine.vi"("State(s) in (\"\")"=w222) -> ("States Out"=w221:string)  [unwired: 14 in]
      }
      frame "UI: Bring Window to Topmost(Windows Only)" {
        n94 = disable-structure shown="OS==Win" {
          disable-tunnel: [w235 _] -> w228
          disable-tunnel: w227 -> [w234 _]
          frame condition #0 (active) {
            w240 = 0 items=["NULL"]
            # "How to Bring the Front Panel in Front of All Desktop Windows? -Batch File Method\nhttps://knowledge.ni.com/KnowledgeArticleDetails?id=kA03q000000YOu6CAG&l=en-US"
            n95 = Unbundle By Name(w234) -> ("Core.Current VI Reference"=w233:refnum<vi>)
            n96 = property class="VI"(reference=w233) -> (error out=w236:errorcluster, "Front Panel.Title"=w237:string)  [unwired: 1 in, 1 out]
            n97 = call "CSM - user.lib Dir.vi"() -> ("csm_user.lib_dir"=w232:path)  [unwired: 2 in, 1 out]
            n98 = dll-call lib="user32.dll" fn="FindWindowA" label="FindWindow"(error in=w236, "lpszClassName"=w240, "lpszWindowName"=w237) -> (error out=w239:errorcluster, "hWnd"=w238:u64)  [unwired: 3 in, 2 out]
            n99 = Build Path(base path=w232, name or relative path=path "_scripts/sendkeys.bat") -> (appended path=w230:path)
            n100 = case shown="Default" w238 {
              selector: w238 -> [_ w247]
              tunnel: w239 -> [w241 w248]
              tunnel: [w241 w246] -> w235
              tunnel: w230 -> [_ w244]
              frame 0 {
              }
              frame Default {
                n101 = dll-call lib="user32.dll" fn="SetForegroundWindow"(error in=w248, "Handle"=w247) -> (error out=w245:errorcluster)  [unwired: 3 in, 2 out]
                n102 = call <vilib>:"Check if File or Folder Exists.vi"("path"=w244) -> ("file or folder exists?"=w242:bool, "dup path"=w243:path)  [unwired: 8 in, 1 out]
                n103 = case shown="True" w242 {
                  tunnel: [w249 w254] -> w246
                  tunnel: w245 -> [w249 w253]
                  tunnel: w243 -> [_ w250]
                  frame False {
                  }
                  frame True {
                    n104 = Format Into String(format string="\"%s\" \"LabVIEW\" \"\"" ("command line"), w250) -> (resulting string=w251:string)  [unwired: 2 in, 1 out]
                    n105 = call <vilib>:"System Exec.vi"("run minimized? (F)"=TRUE, "wait until completion? (T)"=TRUE, "error in (no error)"=w253, "command line"=w251) -> ("error out"=w254:errorcluster)  [unwired: 4 in, 3 out]
                  }
                }
              }
            }
          }
          frame condition #1 {
          }
        }
      }
      frame "UI: Front Panel State" {
        # "Argument"
        # "Set Front Panel Open or Closed\n(Usage: \"UI: Front Panel State >> Open|Close\")"
        n106 = Unbundle By Name(w259) -> ("Core.Current VI Reference"=w258:refnum<vi>)
        n107 = case shown="\"Minimize\", \"Minimized\"" w257 {
          tunnel: w261 -> [w269 w284 w295 w308 w321]
          tunnel: [w271 w285 w297 w310 w323] -> w260
          tunnel: w258 -> [w270 w282 w296 w309 w322]
          frame "Open", "Standard", Default {
            w264 = T1."Standard" ("State")
            n108 = property class="VI"(reference=w270, error in=w269) -> (reference out=w267:refnum<vi>, error out=w268:errorcluster, "FP.State"=w266:T1)
            n109 = Not Equal?(x=w266, y=w264) -> (x != y?=w265:bool)
            n110 = case shown="True" w265 {
              tunnel: [w275 w277] -> w271
              tunnel: w268 -> [w274 w277]
              tunnel: w267 -> [w273 _]
              tunnel: w264 -> [w272 _]
              frame True {
                n111 = invoke class="VI" method="FP.Open"(reference=w273, error in=w274, "Activate"=TRUE, "State"=w272) -> (error out=w275:errorcluster)  [unwired: 1 in, 4 out]
              }
              frame False {
              }
            }
          }
          frame "Close", "Closed" {
            n112 = property class="VI"(reference=w282, error in=w284) -> (reference out=w281:refnum<vi>, error out=w283:errorcluster, "FP.State"=w279:T1)
            n113 = Not Equal?(x=w279, y=T1."Closed" ("Front Panel Window:State")) -> (x != y?=w278:bool)
            n114 = case shown="True" w278 {
              tunnel: [w286 w289] -> w285
              tunnel: w283 -> [w286 w288]
              tunnel: w281 -> [_ w287]
              frame False {
              }
              frame True {
                n115 = invoke class="VI" method="FP.Close"(reference=w287, error in=w288) -> (error out=w289:errorcluster)  [unwired: 1 in, 2 out]
              }
            }
          }
          frame "Hidden", "Hide" {
            w290 = T1."Hidden" ("State")
            n116 = property class="VI"(reference=w296, error in=w295) -> (reference out=w293:refnum<vi>, error out=w294:errorcluster, "FP.State"=w292:T1)
            n117 = Not Equal?(x=w292, y=w290) -> (x != y?=w291:bool)
            n118 = case shown="True" w291 {
              tunnel: [w301 w302] -> w297
              tunnel: w294 -> [w300 w302]
              tunnel: w293 -> [w299 _]
              tunnel: w290 -> [w298 _]
              frame True {
                n119 = invoke class="VI" method="FP.Open"(reference=w299, error in=w300, "State"=w298) -> (error out=w301:errorcluster)  [unwired: 2 in, 4 out]
              }
              frame False {
              }
            }
          }
          frame "Minimize", "Minimized" {
            w303 = T1."Minimized" ("State")
            n120 = property class="VI"(reference=w309, error in=w308) -> (reference out=w306:refnum<vi>, error out=w307:errorcluster, "FP.State"=w305:T1)
            n121 = Not Equal?(x=w305, y=w303) -> (x != y?=w304:bool)
            n122 = case shown="True" w304 {
              tunnel: [w314 w315] -> w310
              tunnel: w307 -> [w313 w315]
              tunnel: w306 -> [w312 _]
              tunnel: w303 -> [w311 _]
              frame True {
                n123 = invoke class="VI" method="FP.Open"(reference=w312, error in=w313, "State"=w311) -> (error out=w314:errorcluster)  [unwired: 2 in, 4 out]
              }
              frame False {
              }
            }
          }
          frame "Maximize", "Maximized" {
            w316 = T1."Maximized" ("State")
            n124 = property class="VI"(reference=w322, error in=w321) -> (reference out=w319:refnum<vi>, error out=w320:errorcluster, "FP.State"=w318:T1)
            n125 = Not Equal?(x=w318, y=w316) -> (x != y?=w317:bool)
            n126 = case shown="True" w317 {
              tunnel: [w327 w328] -> w323
              tunnel: w320 -> [w326 w328]
              tunnel: w319 -> [w325 _]
              tunnel: w316 -> [w324 _]
              frame True {
                n127 = invoke class="VI" method="FP.Open"(reference=w325, error in=w326, "State"=w324) -> (error out=w327:errorcluster)  [unwired: 2 in, 4 out]
              }
              frame False {
              }
            }
          }
        }
        n128 = call <vilib>:"Add State(s) to Queue__JKI_lib_State_Machine.vi"("State(s) in (\"\")"=w263) -> ("States Out"=w262:string)  [unwired: 14 in]
      }
      frame "UI: Post Action" {
        n129 = Unbundle By Name(w339) -> ("Polish.Hold"=w337:bool, "Polish.2D Picture"=w335:refnum<vi>, "Polish.Slides"=w334:picture[], "Polish.Action"=w342:refnum<vi>, "Polish.Progress Bar"=w344:refnum<vi>)
        n130 = property on="Property Node" class="LstBox (strict)"(reference=w346) -> (reference out=w348:refnum<vi>, error out=w347:errorcluster, "Value"=w338:i32, "Item Symbols"=w356:i32[], "Item Names"=w345:string[])  [unwired: 1 in]
        n131 = call "Periodic Trigger (OpenG).vi"("Time (ms)"=u32 3000 ("time (ms)")) -> ("Triggered"=w332:bool)  [unwired: 12 in, 2 out]
        n132 = Not(x=w337) -> (.not. x?=w340:bool)
        n133 = And(x=w332, y=w340) -> (x .and. y?=w336:bool)
        n134 = case shown="True" w336 {
          tunnel: w335 -> [_ w366]
          tunnel: w334 -> [_ w362]
          frame False {
          }
          frame True {
            n135 = property class="Pict"(reference=w366) -> (reference out=w361:refnum<vi>, "Value"=w365:picture)  [unwired: 1 in, 1 out]
            n136 = Array Size(array=w362) -> (size(s)=w358:i32)
            n137 = Search 1D Array(1D array=w362, element=w365) -> (index of element=w364:i32)  [unwired: 1 in]
            n138 = Increment(x=w364) -> (x+1=w359:i32)
            n139 = Quotient & Remainder(x=w359, y=w358) -> (x-y*floor(x/y)=w363:i32)  [unwired: 1 out]
            n140 = Index Array(array=w362, index=w363) -> (element=w360:picture)
            n141 = property class="Pict"(reference=w361, "Value"=w360) -> ()  [unwired: 1 in, 2 out]
          }
        }
        n142 = Replace Array Subset(array=w356, new element=1 ("new element/subarray"), index=w338) -> (w354:i32[])
        n143 = Subtract(x=w338, y=5) -> (x-y=w351:i32)
        n144 = Increment(x=w338) -> (x+1=w343:i32)
        n145 = Increment(x=w338) -> (x+1=w329:i32)
        n146 = Increment(x=w338) -> (x+1=w353:i32)
        n147 = property class="Slide (strict)"(reference=w344, "Value"=w343) -> ()  [unwired: 1 in, 2 out]
        n148 = Max & Min(x=w351, y=0) -> (max(x,y)=w349:i32)  [unwired: 1 out]
        n149 = Index Array(array=w345, index=w329) -> (element=w341:string)
        n150 = property on="Property Node" class="LstBox (strict)"(reference=w348, error in=w347, "Top Row"=w349, "Item Symbols"=w354, "Value"=w353) -> ()  [unwired: 2 out]
        n151 = property class="Str"(reference=w342, "Value"=w341) -> ()  [unwired: 1 in, 2 out]
        n152 = call <vilib>:"Add State(s) to Queue__JKI_lib_State_Machine.vi"("State(s) in (\"\")"=w330) -> ("States Out"=w331:string)  [unwired: 14 in]
      }
      frame "---------- Macro ----------" {
        # "Do not put any code in this frame.\n(It is a separator no-op. You can make a copy of this frame to create a new Macro frame)"
        n153 = call <vilib>:"Add State(s) to Queue__JKI_lib_State_Machine.vi"("State(s) in (\"\")"=w370) -> ("States Out"=w369:string)  [unwired: 14 in]
      }
      frame "Macro: Initialize" {
        # "Initialization Macro\n(This is called once, when the VI starts)"
        n154 = call <vilib>:"Add State(s) to Queue__JKI_lib_State_Machine.vi"("State(s) in Front (\"\")"="Data: Initialize\nData: InitializePolish\nInitialize Core Data\nData: List all lvclasses\nData: List all _JKI State Machine Helper VIs\nData: List all _JKI State Machine Helper Folders\nData: List all CSM Templates\nUI: Initialize\nUI: Front Panel State >> Open\nUI: Bring Window to Topmost(Windows Only)\nInitialize: Append steps of fixing JKISM Editor in MultiListbox\nInitialize: Append Simplify lvclass steps in Multilistbox\n//UI: Append Item to Multilistbox >> Refersh More Template palette\n//Initialize: Append Mass Compile Steps in MultiListbox\nInitialize: Append steps of et_csm_doc_case_as_default\n//github #330 https://github.com/NEVSTOP-LAB/Communicable-State-Machine/issues/330\n//Macro: Localize CSM\nMacro: Open VI for recompile\nInsert Task >> Refresh Popup Menus\nUI: Refresh Listbox\nMacro: Set Toolbar Entry Run when Opened\n\n//---------------\nMacro: Start\n//---------------\nMacro: Exit", "State(s) in (\"\")"=w375) -> ("States Out"=w374:string)  [unwired: 13 in]
      }
      frame "Macro: Start" {
        n155 = Unbundle By Name(w380) -> ("Actions"=w379:string[])
        n156 = call "CSM - Compact Multiple States.vi"("Multiple States"=w379) -> ("States"=w376:string)  [unwired: 9 in]
        n157 = call <vilib>:"Add State(s) to Queue__JKI_lib_State_Machine.vi"("State(s) in Front (\"\")"=w376, "State(s) in (\"\")"=w377) -> ("States Out"=w378:string)  [unwired: 13 in]
      }
      frame "Macro: Open VI for recompile" {
        n158 = Build Array("_xnode" ("name or relative path"), "_csmHelper" ("name or relative path"), "_popupMenuPlugin" ("name or relative path"), "_tool" ("name or relative path")) -> (w388:string[])
        n159 = for {
          tunnel: w388 -> [w404] mode=indexing
          tunnel: [w395] -> w389 mode=concatenating
          w396 = TRUE ("Treat LLBs as Folders?")
          n160 = call "CSM - user.lib Dir.vi"() -> ("csm_user.lib_dir"=w402:path)  [unwired: 2 in, 1 out]
          n161 = Build Path(base path=w402, name or relative path=w404) -> (appended path=w403:path)
          n162 = Path To String(path=w402) -> (string=w401:string)
          n163 = String Length(string=w401) -> (length=w400:i32)
          n164 = call <vilib>:"Recursive File List.vi"("pattern"="*.vi", "Continue Recursing on Error? (F)"=w396, "Treat LLBs as Folders?"=w396, "Folder Path"=w403) -> ("All Files in Dir"=w397:path[])  [unwired: 3 in, 4 out]
          n165 = for {
            tunnel: w397 -> [w412] mode=indexing
            tunnel: w400 -> [w410]
            tunnel: [w405] -> w398 mode=indexing
            n166 = Path To String(path=w412) -> (string=w411:string)
            n167 = String Subset(string=w411, offset (0)=w410) -> (substring=w409:string)  [unwired: 1 in]
            n168 = call <vilib>:"Build State String with Arguments__JKI_lib_State_Machine.vi"("Arguments (\"\")"=w409, "State"="Open VIRef to Compile CSM Tools") -> ("State with Arguments"=w407:string)  [unwired: 4 in]
            n169 = call <vilib>:"Build State String with Arguments__JKI_lib_State_Machine.vi"("Arguments (\"\")"=w407, "State"="Insert Task") -> ("State with Arguments"=w405:string)  [unwired: 4 in]
          }
          n170 = Reverse 1D Array(array=w398) -> (reversed array=w395:string[])
        }
        n171 = call "CSM - Compact Multiple States.vi"("Multiple States"=w389) -> ("States"=w385:string)  [unwired: 9 in]
        n172 = call <vilib>:"Add State(s) to Queue__JKI_lib_State_Machine.vi"("State(s) in (\"\")"="UI: Bring Window to Topmost(Windows Only)\nInsert Task >> Open VIRef to Compile CSM Tools2  >> user.lib\\_NEVSTOP\\Communicable State Machine(CSM)\\CSM User Interface(UI) Module Template.vi\nInsert Task >> Open VIRef to Compile CSM Tools2 >> user.lib\\_NEVSTOP\\Communicable State Machine(CSM)\\CSM Module Template.vi\nInsert Task >> Open VIRef to Compile CSM Tools2 >> templates\\Communicable State Machine(CSM)\\CSM DQMH-Style Template.vi\nInsert Task >> Open VIRef to Compile CSM Tools2 >> templates\\Communicable State Machine(CSM)\\CSM Module Template - Tiny.vi\nInsert Task >> Open VIRef to Compile CSM Tools2 >> templates\\Communicable State Machine(CSM)\\CSM User Interface(UI) Module Template - Tiny.vi" ("State(s) in Front (\"\")"), "State(s) at Back (\"\")"=w385) -> ("States Out"=w386:string)  [unwired: 13 in]
        n173 = call <vilib>:"Add State(s) to Queue__JKI_lib_State_Machine.vi"("State(s) in Front (\"\")"=w386, "State(s) in (\"\")"=w391) -> ("States Out"=w392:string)  [unwired: 13 in]
      }
      frame "Macro: Run CSM to Recompile" {
        n174 = call <vilib>:"Add State(s) to Queue__JKI_lib_State_Machine.vi"("State(s) in (\"\")"="Insert Task >> Run Template to Compile CSM API >> user.lib\\_NEVSTOP\\Communicable State Machine(CSM)\\CSM User Interface(UI) Module Template.vi\nInsert Task >> Run Template to Compile CSM API >> user.lib\\_NEVSTOP\\Communicable State Machine(CSM)\\CSM Module Template.vi\nInsert Task >> Run Template to Compile CSM API >> templates\\Communicable State Machine(CSM)\\CSM DQMH-Style Template.vi\nInsert Task >> Run Template to Compile CSM API >> templates\\Communicable State Machine(CSM)\\CSM Module Template - Tiny.vi\nInsert Task >> Run Template to Compile CSM API >> templates\\Communicable State Machine(CSM)\\CSM User Interface(UI) Module Template - Tiny.vi" ("State(s) in Front (\"\")")) -> ("States Out"=w413:string)  [unwired: 14 in]
        n175 = call <vilib>:"Add State(s) to Queue__JKI_lib_State_Machine.vi"("State(s) in Front (\"\")"=w413, "State(s) in (\"\")"=w415) -> ("States Out"=w416:string)  [unwired: 13 in]
      }
      frame "Macro: Localize CSM" {
        n176 = call <vilib>:"Add State(s) to Queue__JKI_lib_State_Machine.vi"("State(s) in (\"\")"="//Insert Task >> Check System Language\n//Insert Task >> Load Localization Files\n//Initialize: Localize All VIs\n//UI: Bring Window to Topmost(Windows Only)" ("State(s) in Front (\"\")")) -> ("States Out"=w419:string)  [unwired: 14 in]
        n177 = call <vilib>:"Add State(s) to Queue__JKI_lib_State_Machine.vi"("State(s) in Front (\"\")"=w419, "State(s) in (\"\")"=w421) -> ("States Out"=w422:string)  [unwired: 13 in]
      }
      frame "Macro: Set Toolbar Entry Run when Opened" {
        n178 = call "_script_enable_run_when_opened.vi"() -> ("error out"=w425:errorcluster)  [unwired: 11 in]
        n179 = call <vilib>:"Clear Errors.vi"("error in (no error)"=w425) -> ()  [unwired: 5 in, 2 out]
      }
      frame "Macro: Exit" {
        # "Exit Macro\n(This is called once, when the VI exits)"
        n180 = Unbundle By Name(w435) -> ("Core.Close Panel on Exit?"=w434:bool)
        n181 = Select(t="UI: Front Panel State >> Close", s=w434, f="") -> (s? t:f=w431:string)
        n182 = call <vilib>:"Add State(s) to Queue__JKI_lib_State_Machine.vi"("State(s) in (\"\")"=w431, "State(s) at Back (\"\")"="Data: Cleanup\nExit") -> ("States Out"=w429:string)  [unwired: 13 in]
        n183 = call <vilib>:"Add State(s) to Queue__JKI_lib_State_Machine.vi"("State(s) in Front (\"\")"=w429, "State(s) in (\"\")"=w438) -> ("States Out"=w437:string)  [unwired: 13 in]
      }
      frame "---------------- Initialize ----------------" {
      }
      frame "Initialize: Append Recompile Steps in MultiListbox" {
        n184 = Unbundle By Name(w449) -> ("Actions"=w443:string[], "_JKI State Machine Helper VIs"=w448:path[])
        n185 = VI Library() -> (path=w446:path)
        n186 = Strip Path(path=w446) -> (stripped path=w445:path)  [unwired: 1 out]
        n187 = for {
          tunnel: w448 -> [w456] mode=indexing
          tunnel: [w452] -> w450 mode=indexing
          tunnel: w445 -> [w455]
          n188 = Path To String(path=w456) -> (string=w454:string)
          n189 = Path To String(path=w455) -> (string=w453:string)
          n190 = Search and Replace String(input string=w454, search string=w453) -> (result string=w457:string)  [unwired: 6 in, 3 out]
          n191 = Format Into String(format string="Recompile >> %s", w457) -> (resulting string=w452:string)  [unwired: 2 in, 1 out]
        }
        n192 = Build Array (concatenate)(w443, w450) -> (w442:string[])
        n193 = Bundle By Name(cluster=w449, "Actions"=w442) -> (w444:T3)
      }
      frame "Initialize: Append steps of fixing JKISM Editor in MultiListbox" {
        n194 = Unbundle By Name(w463) -> ("Actions"=w461:string[])
        n195 = Build Array (concatenate)(w461, string[] ["Fix JKISM Editor: fix_vi broken in Tree__JKI_State_Machine_Helper.vi", "Fix JKISM Editor: fix_Parse State Queue in Find Parse State Queue vi name.vi", "Fix JKISM Editor: fix_Parse State Queue in Find Parse State Queue vi name2.vi", "Fix JKISM Editor: Fix fix_exclude event case ref check.vi", "Fix JKISM Editor: fix_Find Event Stucture Ref vi.vi", "Fix JKISM Editor: fix_list event frames.vi"] ("element")) -> (w460:string[])
        n196 = Bundle By Name(cluster=w463, "Actions"=w460) -> (w462:T3)
      }
      frame "Initialize: Append Simplify lvclass steps in Multilistbox" {
        n197 = Unbundle By Name(w472) -> ("Actions"=w466:string[], "CSM lvclass"=w471:path[])
        n198 = call "CSM - user.lib Dir.vi"() -> ("<LabVIEW>"=w469:path)  [unwired: 2 in, 1 out]
        n199 = for {
          tunnel: w471 -> [w476] mode=indexing
          tunnel: [w481] -> w473 mode=indexing
          tunnel: w469 -> [w475]
          n200 = Path To String(path=w476) -> (string=w479:string)
          n201 = Path To String(path=w475) -> (string=w478:string)
          n202 = Search and Replace String(input string=w479, search string=w478) -> (result string=w477:string)  [unwired: 6 in, 3 out]
          n203 = Format Into String(format string="Clear lvclass mutation history >> %s", w477) -> (resulting string=w481:string)  [unwired: 2 in, 1 out]
        }
        n204 = Build Array (concatenate)(w466, w473) -> (w467:string[])
        n205 = Bundle By Name(cluster=w472, "Actions"=w467) -> (w468:T3)
      }
      frame "Initialize: Append Mass Compile Steps in MultiListbox" {
        n206 = Unbundle By Name(w490) -> ("Actions"=w484:string[], "_JKI State Machine Helper Folders"=w489:path[])
        n207 = VI Library() -> (path=w487:path)
        n208 = Strip Path(path=w487) -> (stripped path=w486:path)  [unwired: 1 out]
        n209 = for {
          tunnel: w489 -> [w496] mode=indexing
          tunnel: [w492] -> w482 mode=indexing
          tunnel: w486 -> [w495]
          n210 = Path To String(path=w496) -> (string=w494:string)
          n211 = Path To String(path=w495) -> (string=w493:string)
          n212 = Search and Replace String(input string=w494, search string=w493) -> (result string=w497:string)  [unwired: 6 in, 3 out]
          n213 = Format Into String(format string="Mass Compile >> %s", w497) -> (resulting string=w492:string)  [unwired: 2 in, 1 out]
        }
        n214 = Build Array (concatenate)(w484, w482) -> (w483:string[])
        n215 = Bundle By Name(cluster=w490, "Actions"=w483) -> (w485:T3)
      }
      frame "Initialize: Append steps of et_csm_doc_case_as_default" {
        n216 = Unbundle By Name(w505) -> ("Actions"=w499:string[], "CSM Templates"=w504:path[])
        n217 = call "CSM - user.lib Dir.vi"() -> ("<LabVIEW>"=w502:path)  [unwired: 2 in, 1 out]
        n218 = for {
          tunnel: w504 -> [w511] mode=indexing
          tunnel: [w508] -> w506 mode=indexing
          tunnel: w502 -> [w510]
          n219 = Path To String(path=w511) -> (string=w513:string)
          n220 = Path To String(path=w510) -> (string=w512:string)
          n221 = Search and Replace String(input string=w513, search string=w512) -> (result string=w509:string)  [unwired: 6 in, 3 out]
          n222 = Format Into String(format string="Set First CSM Case >> %s", w509) -> (resulting string=w508:string)  [unwired: 2 in, 1 out]
        }
        n223 = Build Array (concatenate)(w499, w506) -> (w500:string[])
        n224 = Bundle By Name(cluster=w505, "Actions"=w500) -> (w501:T3)
      }
      frame "Initialize: Append Item to Multilistbox", "Insert Task" {
        n225 = Unbundle By Name(w519) -> ("Actions"=w517:string[])
        n226 = Build Array(w521) -> (w520:string[])
        n227 = Build Array (concatenate)(w517, w520) -> (w516:string[])
        n228 = Bundle By Name(cluster=w519, "Actions"=w516) -> (w518:T3)
      }
      frame "Initialize: Localize All VIs" {
        n229 = call "CSM - user.lib Dir.vi"() -> ("<LabVIEW>"=w526:path)  [unwired: 2 in, 1 out]
        n230 = Unbundle By Name(w534) -> ("Actions"=w530:string[])
        n231 = Path to Array of Strings(0:w526) -> (2:w528:string[])  [unwired: 1 out]
        n232 = call "_list_CSM documented VIs.vi"() -> ("Array"=w529:path[])  [unwired: 11 in]
        n233 = Array Size(array=w528) -> (size(s)=w527:i32)
        n234 = for {
          tunnel: w529 -> [w542] mode=indexing
          tunnel: w527 -> [w540]
          tunnel: [w539] -> w525 mode=indexing
          n235 = Path to Array of Strings(0:w542) -> (2:w541:string[])  [unwired: 1 out]
          n236 = Array Subset(array=w541, index=w540) -> (w538:string[])  [unwired: 1 in]
          n237 = Array of Strings to Path(0:w538, 1:TRUE ("relative")) -> (2:w539:path)
        }
        n238 = Path To String(path=w525) -> (string=w523:string[])
        n239 = for {
          tunnel: [w545] -> w535 mode=indexing
          tunnel: "Localize VI Description >> %s" ("format string") -> [w544]
          tunnel: w523 -> [w543] mode=indexing
          n240 = Format Into String(format string=w544, w543) -> (resulting string=w545:string)  [unwired: 2 in, 1 out]
        }
        n241 = Build Array (concatenate)(w530, w535) -> (w531:string[])
        n242 = Bundle By Name(cluster=w534, "Actions"=w531) -> (w532:T3)
      }
      frame "---------- Action ----------" {
        # "Template Separator\n(You can make a copy of, or modify, this frame)"
        n243 = call <vilib>:"Add State(s) to Queue__JKI_lib_State_Machine.vi"("State(s) in (\"\")"=w549) -> ("States Out"=w548:string)  [unwired: 14 in]
      }
      frame "Recompile" {
        n244 = String To Path(string=w554) -> (path=w553:path)
        n245 = Open VI Reference(vi path=w553) -> (vi reference=w560:refnum<vi>, error out=w561:errorcluster)  [unwired: 5 in]
        n246 = invoke class="VI" method="Compile"(reference=w560, error in=w561, "Entire Hierarchy"=FALSE ("Compile Entire Hierarchy (F)"), "Force Compile"=TRUE ("Force Compile (T)")) -> (reference out=w559:refnum<vi>, error out=w558:errorcluster)  [unwired: 1 in, 3 out]
        n247 = invoke class="VI" method="Save.Instrument"(reference=w559, error in=w558) -> (reference out=w556:refnum<vi>, error out=w557:errorcluster)  [unwired: 4 in, 4 out]
        n248 = Close Reference(reference=w556, error in (no error)=w557) -> (error out=w555:errorcluster)
        n249 = call <vilib>:"Clear Errors.vi"("error in (no error)"=w555) -> ()  [unwired: 5 in, 2 out]
        n250 = call <vilib>:"Add State(s) to Queue__JKI_lib_State_Machine.vi"("State(s) in Front (\"\")"="UI: Post Action" ("State(s) in Front (\"\")"), "State(s) in (\"\")"=w551) -> ("States Out"=w552:string)  [unwired: 13 in]
      }
      frame "Set First CSM Case" {
        n251 = Match Pattern(string=w567, regular expression="^[\\\\]*") -> (before substring=w568:string)  [unwired: 1 in, 3 out]
        n252 = String To Path(string=w568) -> (path=w566:path)
        n253 = call "CSM - user.lib Dir.vi"() -> ("<LabVIEW>"=w571:path)  [unwired: 2 in, 1 out]
        n254 = Build Path(base path=w571, name or relative path=w566) -> (appended path=w570:path)
        n255 = call "_script_set_csm_doc_case_as_default.vi"("Vi Path"=w570) -> ("error out"=w575:errorcluster)  [unwired: 10 in]
        n256 = call <vilib>:"Clear Errors.vi"("error in (no error)"=w575) -> ()  [unwired: 5 in, 2 out]
        n257 = call <vilib>:"Add State(s) to Queue__JKI_lib_State_Machine.vi"("State(s) in Front (\"\")"="UI: Post Action" ("State(s) in Front (\"\")"), "State(s) in (\"\")"=w573) -> ("States Out"=w574:string)  [unwired: 13 in]
      }
      frame "Clear lvclass mutation history" {
        n258 = Match Pattern(string=w579, regular expression="^[\\\\]*") -> (before substring=w580:string)  [unwired: 1 in, 3 out]
        n259 = String To Path(string=w580) -> (path=w578:path)
        n260 = call "CSM - user.lib Dir.vi"() -> ("<LabVIEW>"=w583:path)  [unwired: 2 in, 1 out]
        n261 = Build Path(base path=w583, name or relative path=w578) -> (appended path=w582:path)
        n262 = call "clear the mutation history for the classes.vi"("Path"=w582) -> ()  [unwired: 11 in]
        n263 = call <vilib>:"Add State(s) to Queue__JKI_lib_State_Machine.vi"("State(s) in Front (\"\")"="UI: Post Action" ("State(s) in Front (\"\")"), "State(s) in (\"\")"=w585) -> ("States Out"=w586:string)  [unwired: 13 in]
      }
      frame "Fix JKISM Editor: fix_Parse State Queue in Find Parse State Queue vi name.vi" {
        n264 = call "_script_fix_Parse State Queue in Find Parse State Queue vi name.vi"() -> ()  [unwired: 12 in]
        n265 = call <vilib>:"Add State(s) to Queue__JKI_lib_State_Machine.vi"("State(s) in Front (\"\")"="UI: Post Action" ("State(s) in Front (\"\")"), "State(s) in (\"\")"=w590) -> ("States Out"=w591:string)  [unwired: 13 in]
      }
      frame "Fix JKISM Editor: fix_Parse State Queue in Find Parse State Queue vi name2.vi" {
        n266 = call "_script_fix_Parse State Queue in Find Parse State Queue vi name2.vi"() -> ()  [unwired: 12 in]
        n267 = call <vilib>:"Add State(s) to Queue__JKI_lib_State_Machine.vi"("State(s) in Front (\"\")"="UI: Post Action" ("State(s) in Front (\"\")"), "State(s) in (\"\")"=w595) -> ("States Out"=w596:string)  [unwired: 13 in]
      }
      frame "Fix JKISM Editor: fix_vi broken in Tree__JKI_State_Machine_Helper.vi" {
        n268 = call "_script_fix_vi broken in Tree__JKI_State_Machine_Helper.vi"() -> ()  [unwired: 12 in]
        n269 = call <vilib>:"Add State(s) to Queue__JKI_lib_State_Machine.vi"("State(s) in Front (\"\")"="UI: Post Action" ("State(s) in Front (\"\")"), "State(s) in (\"\")"=w600) -> ("States Out"=w601:string)  [unwired: 13 in]
      }
      frame "Fix JKISM Editor: Fix fix_exclude event case ref check.vi" {
        n270 = call "_script_fix_exclude event case ref check.vi"() -> ()  [unwired: 12 in]
        n271 = call <vilib>:"Add State(s) to Queue__JKI_lib_State_Machine.vi"("State(s) in Front (\"\")"="UI: Post Action" ("State(s) in Front (\"\")"), "State(s) in (\"\")"=w605) -> ("States Out"=w606:string)  [unwired: 13 in]
      }
      frame "Fix JKISM Editor: fix_Find Event Stucture Ref vi.vi" {
        n272 = call "_script_fix_Find Event Stucture Ref vi.vi"() -> ()  [unwired: 12 in]
        n273 = call <vilib>:"Add State(s) to Queue__JKI_lib_State_Machine.vi"("State(s) in Front (\"\")"="UI: Post Action" ("State(s) in Front (\"\")"), "State(s) in (\"\")"=w610) -> ("States Out"=w611:string)  [unwired: 13 in]
      }
      frame "Fix JKISM Editor: fix_list event frames.vi" {
        n274 = call "_script_fix_list event frames.vi"() -> ()  [unwired: 12 in]
        n275 = call <vilib>:"Add State(s) to Queue__JKI_lib_State_Machine.vi"("State(s) in Front (\"\")"="UI: Post Action" ("State(s) in Front (\"\")"), "State(s) in (\"\")"=w615) -> ("States Out"=w616:string)  [unwired: 13 in]
      }
      frame "Mass Compile" {
        n276 = Match Pattern(string=w620, regular expression="^[\\\\]*") -> (before substring=w621:string)  [unwired: 1 in, 3 out]
        n277 = String To Path(string=w621) -> (path=w619:path)
        n278 = call "CSM - user.lib Dir.vi"() -> ("<LabVIEW>"=w624:path)  [unwired: 2 in, 1 out]
        n279 = Build Path(base path=w624, name or relative path=w619) -> (appended path=w623:path)
        n280 = invoke class="App" method="Mass Compile"("Directory to Compile"=w623) -> (error out=w630:errorcluster)  [unwired: 8 in, 8 out]
        n281 = call <vilib>:"Clear Errors.vi"("error in (no error)"=w630) -> ()  [unwired: 5 in, 2 out]
        n282 = Wait (ms)(milliseconds to wait=u32 1000) -> ()  [unwired: 1 out]
        n283 = call <vilib>:"Add State(s) to Queue__JKI_lib_State_Machine.vi"("State(s) in Front (\"\")"="UI: Post Action" ("State(s) in Front (\"\")"), "State(s) in (\"\")"=w626) -> ("States Out"=w627:string)  [unwired: 13 in]
      }
      frame "Run Template to Compile CSM API" {
        n284 = String To Path(string=w634) -> (path=w632:path)
        n285 = call "CSM - user.lib Dir.vi"() -> ("<LabVIEW>"=w633:path)  [unwired: 2 in, 1 out]
        n286 = Build Path(base path=w633, name or relative path=w632) -> (appended path=w637:path)
        n287 = call <vilib>:"Check if File or Folder Exists.vi"("path"=w637) -> ("file or folder exists?"=w635:bool, "dup path"=w636:path)  [unwired: 8 in, 1 out]
        n288 = case shown="True" w635 {
          tunnel: w636 -> [w643 w646]
          frame False {
            n289 = Path To String(path=w643) -> (string=w644:string)
            n290 = Two Button Dialog(message=w644, 2:"Ack" ("T button name (\"OK\")")) -> ()  [unwired: 1 in, 1 out]
          }
          frame True {
            n291 = call "uuid.vi"() -> ("UUID"=w649:string)  [unwired: 11 in]
            n292 = Open VI Reference(type specifier VI Refnum (for type only)=refnum<vi> refnum, vi path=w646, options=128) -> (vi reference=w653:refnum<vi>, error out=w654:errorcluster)  [unwired: 3 in]
            n293 = call-by-ref "Start Asynchronous Call"(reference=w653, error in=w654, "Name(\"\" to use uuid)"=w649) -> (reference out=w656:refnum<vi>, error out=w655:errorcluster)  [unwired: 11 in]
            n294 = Close Reference(reference=w656, error in (no error)=w655) -> (error out=w651:errorcluster)
            n295 = flat-sequence {
              tunnel: w651 -> [w658]
              tunnel: [w658] -> w650
              frame #0 {
                n296 = Wait (ms)(milliseconds to wait=u32 500) -> ()  [unwired: 1 out]
              }
            }
            n297 = call "CSM - Send Message and Wait for Reply.vi"("Error In (No Error)"=w650, "Target Module"=w649, "State"="Macro: Exit") -> ("error out"=w647:errorcluster)  [unwired: 6 in, 2 out]
            n298 = call <vilib>:"Clear Errors.vi"("error in (no error)"=w647) -> ()  [unwired: 5 in, 2 out]
          }
        }
        n299 = call <vilib>:"Add State(s) to Queue__JKI_lib_State_Machine.vi"("State(s) in Front (\"\")"="UI: Post Action" ("State(s) in Front (\"\")"), "State(s) in (\"\")"=w639) -> ("States Out"=w640:string)  [unwired: 13 in]
      }
      frame "Open VIRef to Compile CSM Tools" {
        n300 = Match Pattern(string=w663, regular expression="^[\\\\]*") -> (after substring=w661:string)  [unwired: 1 in, 3 out]
        n301 = call "CSM - user.lib Dir.vi"() -> ("csm_user.lib_dir"=w667:path)  [unwired: 2 in, 1 out]
        n302 = String To Path(string=w661) -> (path=w660:path)
        n303 = Build Path(base path=w667, name or relative path=w660) -> (appended path=w668:path)
        n304 = call <vilib>:"Check if File or Folder Exists.vi"("path"=w668) -> ("error out"=w666:errorcluster, "file or folder exists?"=w665:bool, "dup path"=w664:path)  [unwired: 8 in]
        n305 = case shown="True" w665 {
          tunnel: w666 -> [_ w679]
          tunnel: w664 -> [w675 w678]
          frame False {
            n306 = Path To String(path=w675) -> (string=w674:string)
            n307 = Two Button Dialog(message=w674, 2:"Ack" ("T button name (\"OK\")")) -> ()  [unwired: 1 in, 1 out]
          }
          frame True {
            n308 = Open VI Reference(vi path=w678, options=2, error in (no error)=w679) -> (vi reference=w680:refnum<vi>, error out=w684:errorcluster)  [unwired: 3 in]
            n309 = flat-sequence {
              tunnel: w684 -> [w688]
              tunnel: [w687] -> w683
              tunnel: [w685] -> w681
              tunnel: w680 -> [w686]
              frame #0 {
                n310 = invoke class="VI" method="Save.Instrument"(reference=w686, error in=w688) -> (reference out=w685:refnum<vi>, error out=w687:errorcluster)  [unwired: 4 in, 4 out]
                n311 = Wait (ms)(milliseconds to wait=u32 50) -> ()  [unwired: 1 out]
              }
            }
            n312 = Close Reference(reference=w681, error in (no error)=w683) -> (error out=w682:errorcluster)
            n313 = call <vilib>:"Clear Errors.vi"("error in (no error)"=w682) -> ()  [unwired: 5 in, 2 out]
          }
        }
        n314 = call <vilib>:"Add State(s) to Queue__JKI_lib_State_Machine.vi"("State(s) in Front (\"\")"="UI: Post Action" ("State(s) in Front (\"\")"), "State(s) in (\"\")"=w670) -> ("States Out"=w671:string)  [unwired: 13 in]
      }
      frame "Open VIRef to Compile CSM Tools2" {
        n315 = Match Pattern(string=w694, regular expression="^[\\\\]*") -> (after substring=w692:string)  [unwired: 1 in, 3 out]
        n316 = String To Path(string=w692) -> (path=w690:path)
        n317 = call "CSM - user.lib Dir.vi"() -> ("<LabVIEW>"=w691:path)  [unwired: 2 in, 1 out]
        n318 = Build Path(base path=w691, name or relative path=w690) -> (appended path=w698:path)
        n319 = call <vilib>:"Check if File or Folder Exists.vi"("path"=w698) -> ("error out"=w697:errorcluster, "file or folder exists?"=w696:bool, "dup path"=w695:path)  [unwired: 8 in]
        n320 = case shown="True" w696 {
          tunnel: w697 -> [_ w709]
          tunnel: w695 -> [w705 w708]
          frame False {
            n321 = Path To String(path=w705) -> (string=w704:string)
            n322 = Two Button Dialog(message=w704, 2:"Ack" ("T button name (\"OK\")")) -> ()  [unwired: 1 in, 1 out]
          }
          frame True {
            n323 = Open VI Reference(vi path=w708, options=2, error in (no error)=w709) -> (vi reference=w710:refnum<vi>, error out=w714:errorcluster)  [unwired: 3 in]
            n324 = flat-sequence {
              tunnel: w714 -> [w718]
              tunnel: [w717] -> w713
              tunnel: [w715] -> w711
              tunnel: w710 -> [w716]
              frame #0 {
                n325 = invoke class="VI" method="Save.Instrument"(reference=w716, error in=w718) -> (reference out=w715:refnum<vi>, error out=w717:errorcluster)  [unwired: 4 in, 4 out]
                n326 = Wait (ms)(milliseconds to wait=u32 50) -> ()  [unwired: 1 out]
              }
            }
            n327 = Close Reference(reference=w711, error in (no error)=w713) -> (error out=w712:errorcluster)
            n328 = call <vilib>:"Clear Errors.vi"("error in (no error)"=w712) -> ()  [unwired: 5 in, 2 out]
          }
        }
        n329 = call <vilib>:"Add State(s) to Queue__JKI_lib_State_Machine.vi"("State(s) in Front (\"\")"="UI: Post Action" ("State(s) in Front (\"\")"), "State(s) in (\"\")"=w700) -> ("States Out"=w701:string)  [unwired: 13 in]
      }
      frame "Refresh Popup Menus" {
        n330 = VI Library() -> (path=w729:path)
        n331 = Strip Path(path=w729) -> (stripped path=w728:path)  [unwired: 1 out]
        n332 = String To Path(string="resource\\plugins\\PopupMenus\\support\\Refresh Menus.vi" ("name or relative path")) -> (path=w720:path)
        n333 = Build Path(base path=w728, name or relative path=w720) -> (appended path=w726:path)
        n334 = call <vilib>:"Check if File or Folder Exists.vi"("path"=w726) -> ("file or folder exists?"=w724:bool, "dup path"=w725:path)  [unwired: 8 in, 1 out]
        n335 = case shown="True" w724 {
          tunnel: w725 -> [_ w738]
          frame False {
          }
          frame True {
            n336 = Open VI Reference(vi path=w738) -> (vi reference=w737:refnum<vi>, error out=w736:errorcluster)  [unwired: 5 in]
            n337 = invoke class="VI" method="Run VI"(reference=w737, error in=w736, "Wait until done"=TRUE ("Wait Until Done"), "Auto Dispose Ref"=FALSE ("Auto Dispose Reference")) -> (reference out=w732:refnum<vi>, error out=w733:errorcluster)  [unwired: 1 in, 3 out]
            n338 = Close Reference(reference=w732, error in (no error)=w733) -> ()  [unwired: 1 out]
          }
        }
        n339 = call <vilib>:"Add State(s) to Queue__JKI_lib_State_Machine.vi"("State(s) in Front (\"\")"="UI: Post Action" ("State(s) in Front (\"\")"), "State(s) in (\"\")"=w722) -> ("States Out"=w723:string)  [unwired: 13 in]
      }
      frame "Check System Language" {
        n340 = call "_csm_System_Language.vi"() -> ("LangID"=w742:string)  [unwired: 11 in]
        n341 = Bundle By Name(cluster=w744, "LangID"=w742) -> (w743:T3)
        n342 = call <vilib>:"Add State(s) to Queue__JKI_lib_State_Machine.vi"("State(s) in Front (\"\")"="UI: Post Action" ("State(s) in Front (\"\")"), "State(s) in (\"\")"=w740) -> ("States Out"=w741:string)  [unwired: 13 in]
      }
      frame "Load Localization Files" {
        w746 = variant ("DescMap")
        n343 = Unbundle By Name(w751) -> ()  [unwired: 1 out]
        n344 = Bundle By Name(cluster=w751, "DescMap"=w746, "NoteMap"=w746) -> (w750:T3)
        n345 = call <vilib>:"Add State(s) to Queue__JKI_lib_State_Machine.vi"("State(s) in Front (\"\")"="UI: Post Action" ("State(s) in Front (\"\")"), "State(s) in (\"\")"=w748) -> ("States Out"=w749:string)  [unwired: 13 in]
      }
      frame "Localize VI Description" {
        n346 = Unbundle By Name(w760) -> ("LangID"=w761:string, "DescMap"=w763:variant, "NoteMap"=w764:variant)
        n347 = call "CSM - user.lib Dir.vi"() -> ("<LabVIEW>"=w765:path)  [unwired: 2 in, 1 out]
        n348 = Match Pattern(string=w754, regular expression="^[\\\\]*") -> (before substring=w753:string)  [unwired: 1 in, 3 out]
        n349 = Build Path(base path=w765, name or relative path=w753) -> (appended path=w762:path)
        n350 = Strip Path(path=w762) -> (name=w770:string)  [unwired: 1 out]
        n351 = Get Variant Attribute(Variant=w763, name=w770, default value (empty Variant)="" ("String")) -> (found=w769:bool, value=w766:string, error out=w768:errorcluster)  [unwired: 1 in, 1 out]
        n352 = case shown="True" w769 {
          tunnel: w768 -> [w771 w774]
          tunnel: [w771 w775] -> w759
          tunnel: w766 -> [_ w772]
          tunnel: w764 -> [_ _]
          tunnel: w762 -> [_ w773]
          tunnel: w761 -> [_ _]
          frame False {
          }
          frame True {
            n353 = call "Populate Single VI Help.vi"("error in (no error)"=w774, "VI Description"=w772, "Path"=w773) -> ("error out"=w775:errorcluster)  [unwired: 8 in]
          }
        }
        n354 = call <vilib>:"Add State(s) to Queue__JKI_lib_State_Machine.vi"("State(s) in Front (\"\")"="UI: Post Action" ("State(s) in Front (\"\")"), "State(s) in (\"\")"=w757) -> ("States Out"=w758:string)  [unwired: 13 in]
      }
    }
  }
  n355 = call <vilib>:"Clear Errors.vi"("error in (no error)"=w1) -> ()  [unwired: 5 in, 2 out]
